vi "STD Cal Data_etc_old.vi"(8 "error in":errorcluster caption="에러 입력(에러 없음)", 9 "Data in":string[][](array[string]), 10 "문자열":string, 11 "Func_ext":string) -> (0 "error out":errorcluster caption="에러 출력", 1 "Data Out":string[][](array[string]), 3 "Func_ext Out":string, 4 "Data Out 2":string[](array[string]), 6 "Cal STD":string[][](array[string]))   [LabVIEW 2020]
uses:
  Support/Controls/Cmd_Var Data IO.ctl
  Support/Controls/Cmd_File path.ctl
  Support/Controls/Cmd_File Type.ctl
  Variables/Global_Cal STD.vi
  Variables/Global_Cal Info.vi
  Support/Public/Polymorph/Data Class_2D Str.vi
  Support/Public/Polymorph/Sort_2D Str.vi
  Support/Public/Polymorph/Array Dedup_2D Str.vi
  <vilib>/Utility/file.llb/Read Delimited Spreadsheet (string).vi
  Support/Public/Polymorph/Array Dedup_1D Str.vi
panel:
  out "Cal STD in":string[][](array[string])
  out "Condition Default":string[][](array[string])
  out "데이터오류?":bool
  out "생성오류?":bool
  out "Condition":string[][](array[string])
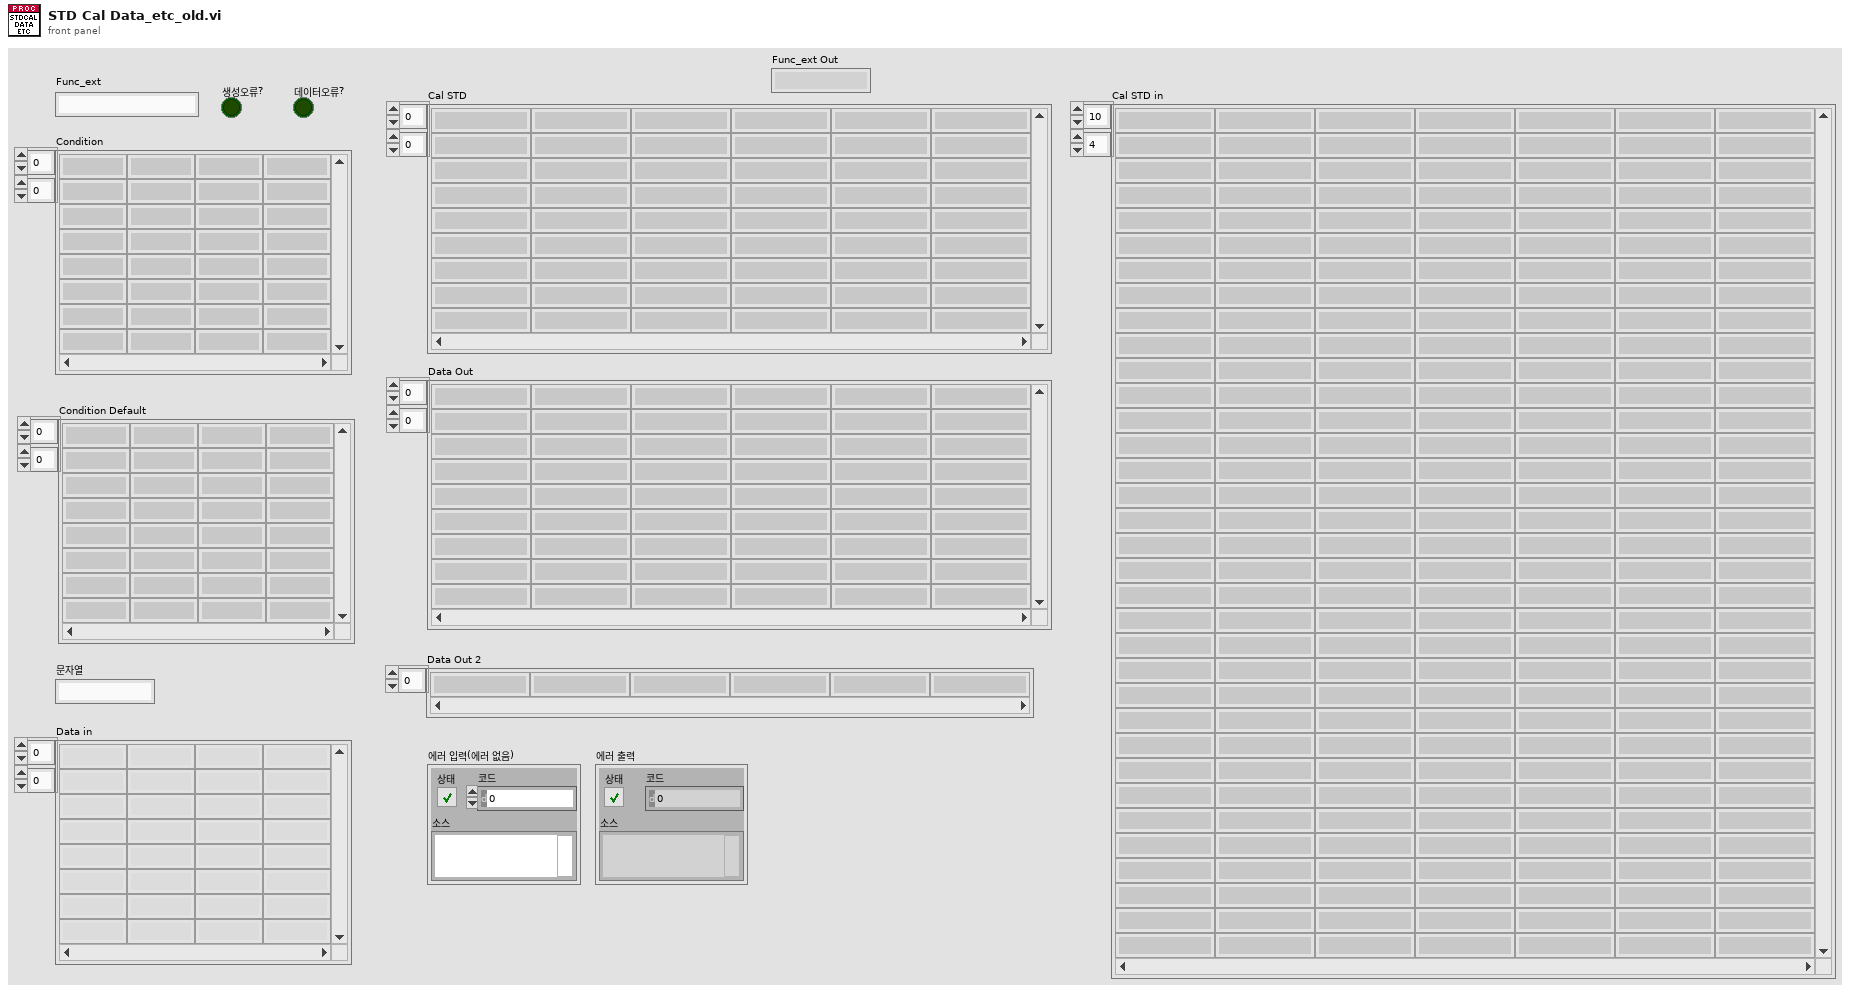
[diagram p1: front panel]
types:
  T1 = typedef "Cmd_Var Data IO.ctl" = enum16{"Condition", "Condition Default", "Condition_Temp", "Resolution", "Resolution Default", "Resolution Old", "Spec", "Spec Default", "Spec Old", "Spec Temp", "Result", "Result2", "Result3", "Result_Temp", "Result_ADJ", "Result_ADJ2", "STD1", "STD2", "STD3", "STD4", "STD5", "STD Temp", "CMC", "CMC Default"}
  T2 = cluster{"세부분류코드":string, "형식":string, "옵션":string, "측정기명":string, "EXCEL파일명":string, "TEMP":string}
  T3 = typedef "Cmd_File Type.ctl" = enum16{"엑셀", "엑셀(2003)", "텍스트", "설정", "2진", "VI", "CSV", "LOG", "폴더"}
  T4 = typedef "Cmd_File path.ctl" = enum16{"에러로그", "데이터파일경로", "성적서원본", "지난성적서", "Data Files", "경로생성", "Updater", "Template", "설정파일경로", "FTP Upload", "Update 경로", "어플리케이션"}
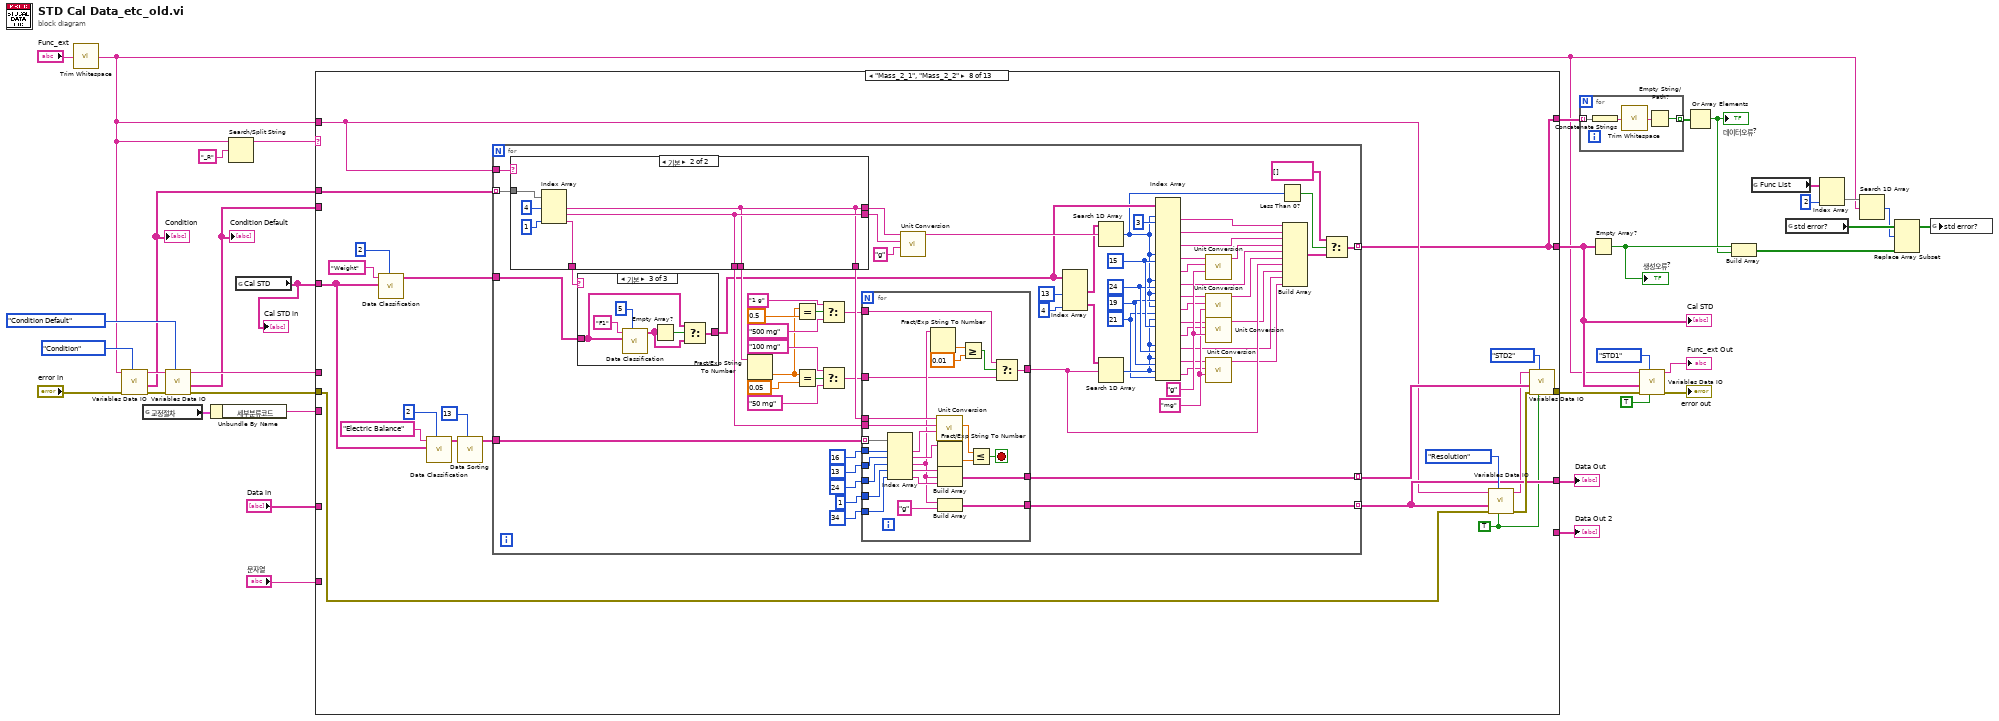
[diagram p0: block diagram]
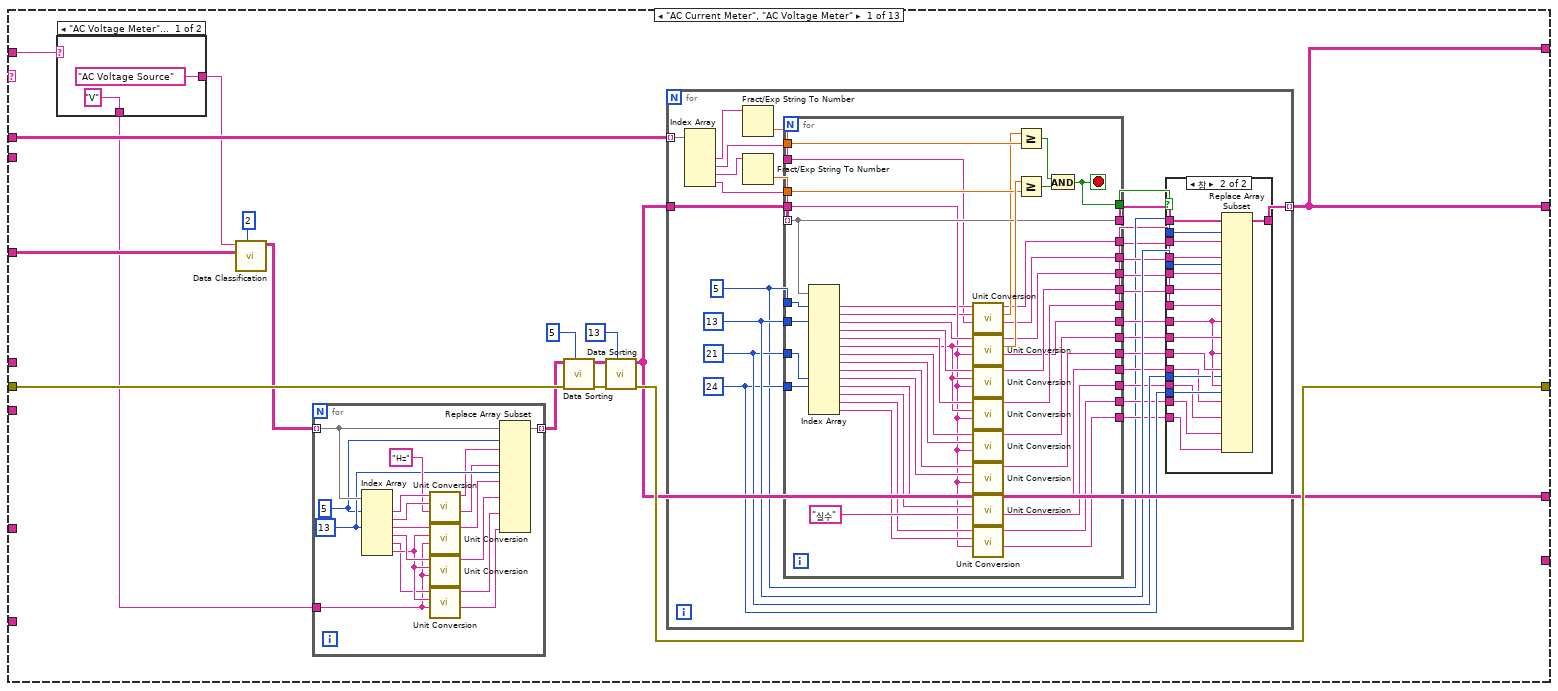
[diagram p2: hidden frame]
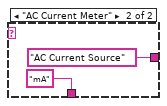
[diagram p3: hidden frame]
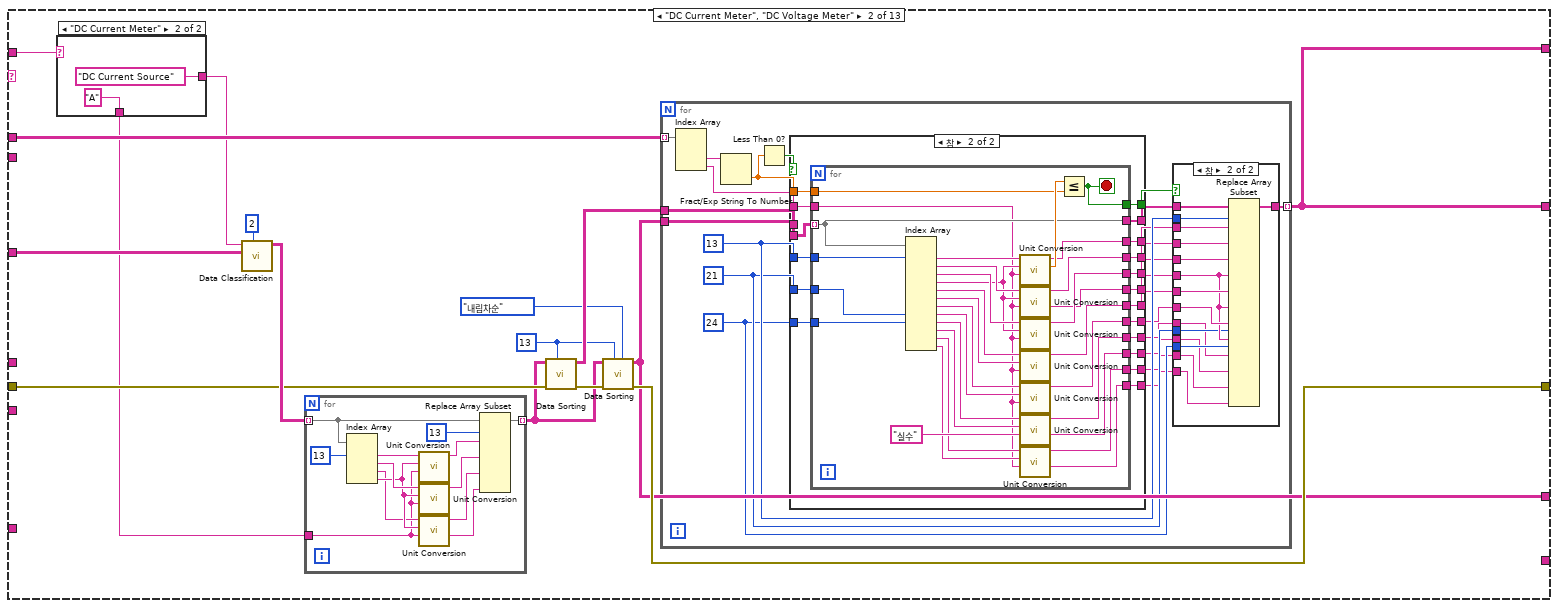
[diagram p5: hidden frame]
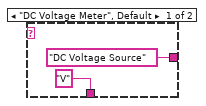
[diagram p6: hidden frame]
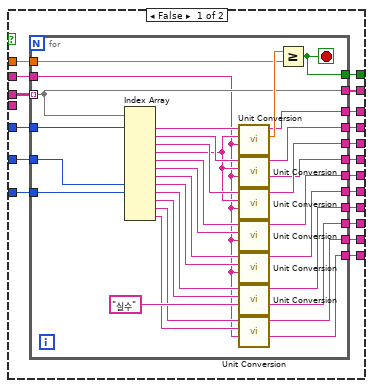
[diagram p8: hidden frame]
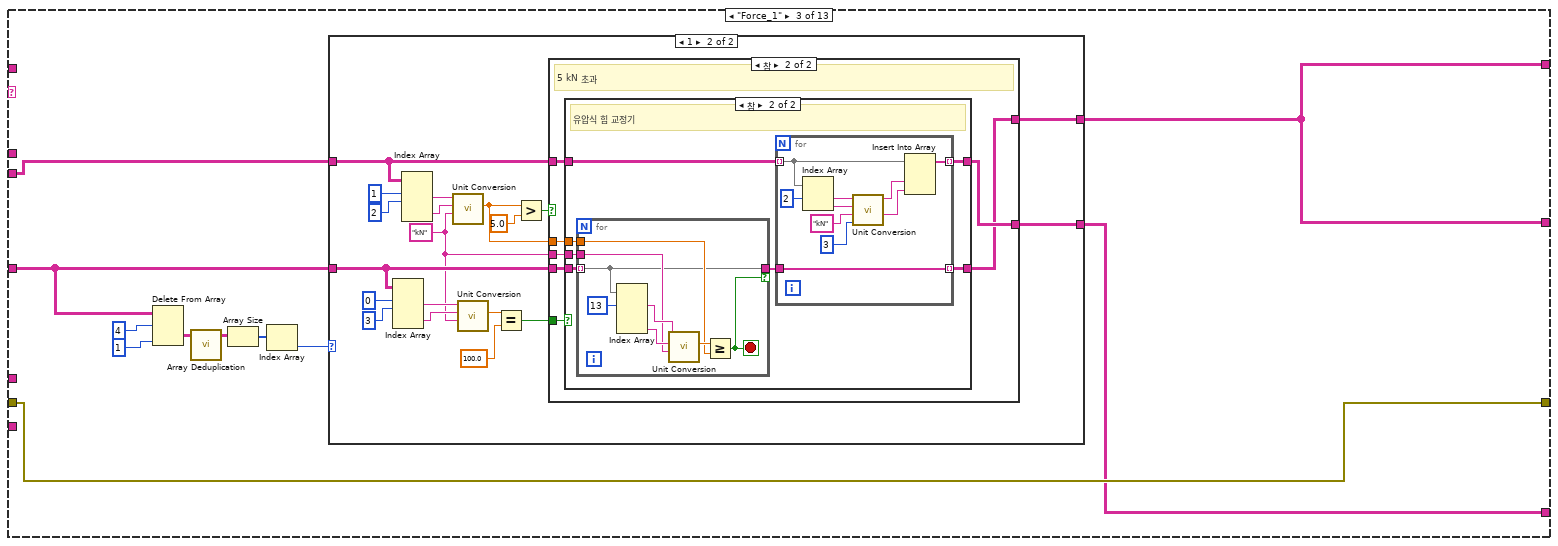
[diagram p9: hidden frame]
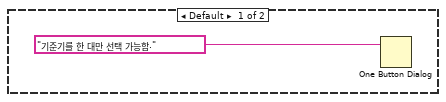
[diagram p10: hidden frame]
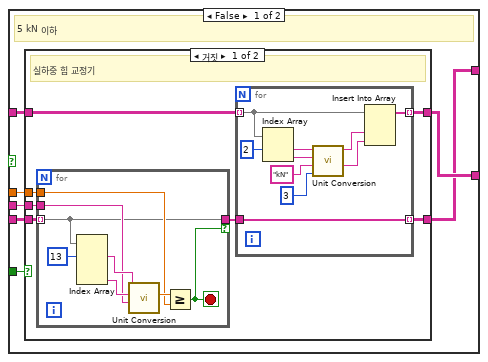
[diagram p11: hidden frame]
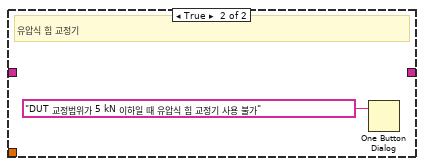
[diagram p12: hidden frame]
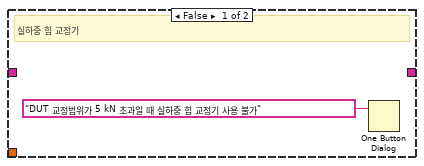
[diagram p13: hidden frame]
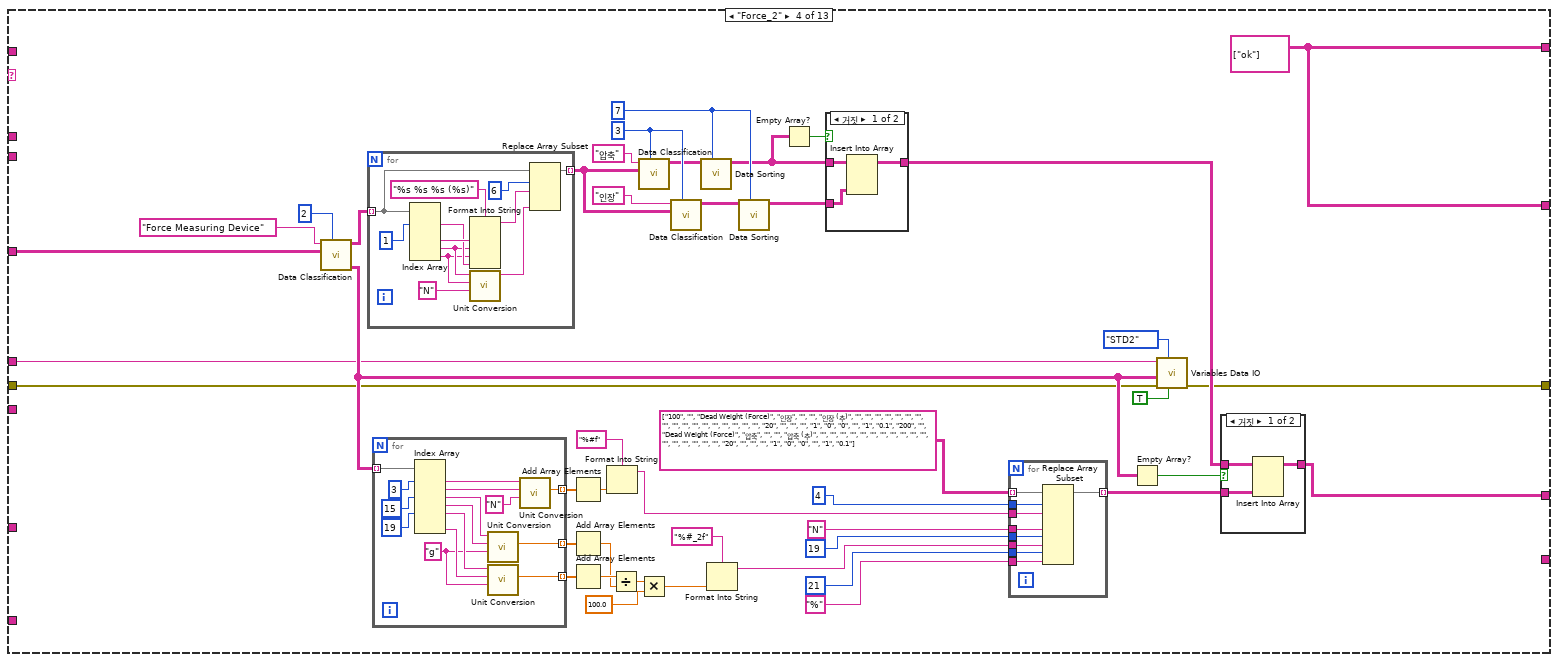
[diagram p14: hidden frame]
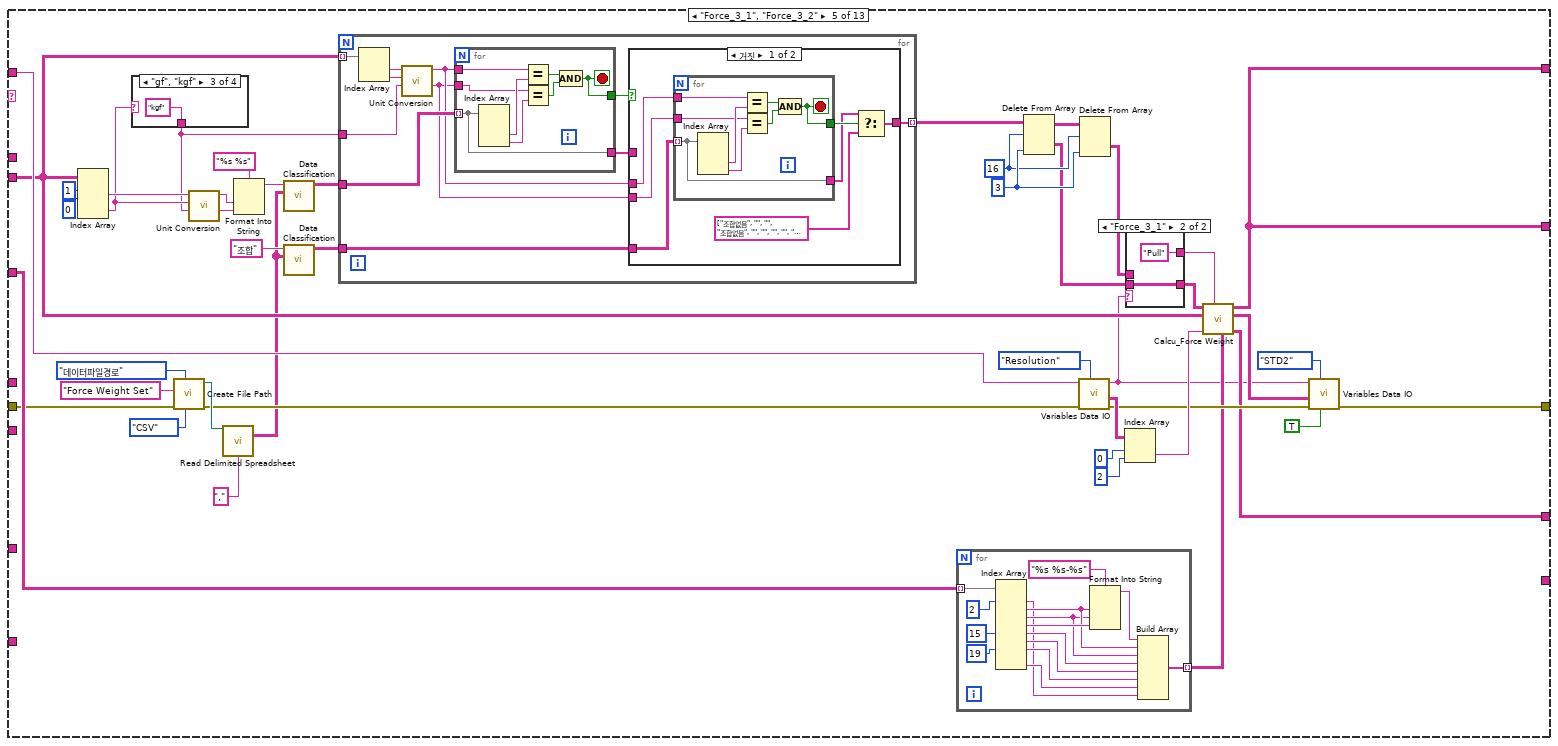
[diagram p17: hidden frame]
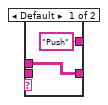
[diagram p18: hidden frame]
diagram:
  n1 = call <vilib>:"Trim Whitespace.vi"("string"="Func_ext") -> ("trimmed string"=w2:string)  [unwired: 1 in]
  n2 = call "Variables Data IO.vi"("Select"=Cmd_Var_Data_IO."Condition", "error in"="error in", "Func_ext"=w2) -> ("error out"=w24:errorcluster, "Data Out"=w9:string[][], "Func_ext Out"=w22:string)  [unwired: 6 in]
  "Condition" <- w9
  n3 = global read "Global_Cal Info.vi" "교정절차"() -> (w7:T2)
  n4 = call "Variables Data IO.vi"("Select"=Cmd_Var_Data_IO."Condition Default", "error in"=w24, "Func_ext"=w22) -> ("error out"=w23:errorcluster, "Data Out"=w8:string[][], "Func_ext Out"=w21:string)  [unwired: 6 in]
  "Condition Default" <- w8
  n5 = Unbundle By Name(w7) -> ("세부분류코드"=w6:string)
  n6 = Search/Split String(string=w2, search string/char (-)="_R" ("검색 문자열/문자 (-)")) -> (substring before match=w19:string)  [unwired: 1 in, 2 out]
  n7 = global read "Global_Cal STD.vi" "Cal STD"() -> (w37:string[][])
  "Cal STD in" <- w37
  n8 = case shown="\"Mass_2_1\", \"Mass_2_2\"" w19 {
    selector: w19 -> [_ _ _ _ _ _ _ _ w978 _ _ _ _]
    tunnel: w23 -> [w48 w174 w341 w442 w517 w628 w718 w852 w986 w1923 w2014 w2127 w2155]
    tunnel: [w50 w170 w341 w447 w533 w626 w738 w853 w984 w1921 w2039 w2126 w2155] -> w36
    tunnel: w37 -> [w52 w176 w334 w463 w551 w629 w754 w856 w983 w1924 w2052 w2128 _]
    tunnel: [w39 w163 w340 w449 w526 w619 w733 w836 w987 w1914 w2033 w2129 w2154] -> w27
    tunnel: [w40 w166 w338 w456 w527 w620 w723 w849 w980 w1915 w2029 w2128 _] -> w33
    tunnel: w9 -> [w51 w173 _ _ _ w627 w713 w847 _ w1922 _ _ _]
    tunnel: [w39 w163 w340 w449 w526 w619 w731 w836 w987 w1914 w2033 w2129 w2154] -> w26
    tunnel: w8 -> [_ _ w339 _ w542 _ _ _ w982 _ w2055 w2125 _]
    tunnel: w21 -> [_ _ _ w445 _ _ _ _ w985 _ w2028 w2124 _]
    tunnel: w2 -> [w38 w162 _ _ w547 w618 w722 w845 _ w1913 _ _ _]
    tunnel: w6 -> [_ _ _ _ _ _ _ _ w981 _ _ _ _]
    tunnel: [_ _ _ _ _ _ _ _ w979 _ _ _ string[] []] -> w5
    tunnel: "Data in" -> [_ _ _ _ _ _ _ _ w976 _ _ _ _]
    tunnel: "문자열" -> [_ _ _ _ _ _ _ _ w977 _ _ _ _]
    frame "AC Current Meter", "AC Voltage Meter" {
      n9 = case shown="\"AC Voltage Meter\", 기본" w38 {
        tunnel: ["AC Voltage Source" "AC Current Source"] -> w42
        tunnel: ["V" ("환산단위") "mA" ("환산단위")] -> w41
        frame "AC Voltage Meter", Default {
        }
        frame "AC Current Meter" {
        }
      }
      n10 = call-poly "Data Classification.vi"("인덱스"=2, "DATA 입력"=w52, "검색 문자열"=w42) -> ("DATA 출력"=w44:string[][])  [unwired: 4 in, 4 out]
      n11 = for {
        tunnel: w44 -> [w160] mode=indexing
        tunnel: [w156] -> w43 mode=indexing
        tunnel: w41 -> [w144]
        w147 = 5 ("인덱스")
        w148 = 13 ("인덱스")
        n12 = Index Array(array=w160, index #1=w147, index #3=w148) -> (element #1=w151:string, element #2=w150:string, element #3=w161:string, element #4=w159:string, element #5=w157:string, element #6=w158:string)  [unwired: 4 in]
        n13 = call "Unit Conversion.vi"("환산단위"="Hz", "입력단위"=w150, "입력값"=w151) -> ("환산단위"=w145:string, "환산값 (string)"=w146:string)  [unwired: 3 in, 4 out]
        n14 = call "Unit Conversion.vi"("환산단위"=w144, "입력단위"=w158, "입력값"=w161) -> ("환산값 (string)"=w155:string)  [unwired: 3 in, 5 out]
        n15 = call "Unit Conversion.vi"("환산단위"=w144, "입력단위"=w158, "입력값"=w159) -> ("환산값 (string)"=w154:string)  [unwired: 3 in, 5 out]
        n16 = call "Unit Conversion.vi"("환산단위"=w144, "입력단위"=w158, "입력값"=w157) -> ("환산단위"=w152:string, "환산값 (string)"=w153:string)  [unwired: 3 in, 4 out]
        n17 = Replace Array Subset(array=w160, new element #1=w146, index #1=w147, new element #2=w145, new element #3=w155, index #3=w148, new element #4=w154, new element #5=w153, new element #6=w152) -> (w156:string[])  [unwired: 4 in]
      }
      n18 = call-poly "Data Sorting.vi"("기준열"=u16 5, "error in (no error)"=w48, "Data in"=w43) -> ("error out"=w47:errorcluster, "Data out"=w46:string[][])  [unwired: 7 in]
      n19 = call-poly "Data Sorting.vi"("기준열"=u16 13, "error in (no error)"=w47, "Data in"=w46) -> ("error out"=w50:errorcluster, "Data out"=w40:string[][])  [unwired: 7 in]
      n20 = for {
        tunnel: w40 -> [w84]
        tunnel: w51 -> [w83] mode=indexing
        tunnel: [w77] -> w39 mode=indexing
        w60 = 5 ("인덱스")
        w74 = 24 ("인덱스")
        w75 = 21 ("인덱스")
        w76 = 13 ("인덱스")
        n21 = Index Array(array=w83) -> (element #2=w63:string, element #3=w61:string, element #4=w80:string, element #5=w82:string)  [unwired: 5 in, 1 out]
        n22 = Fract/Exp String To Number(string=w63) -> (number=w62:dbl)  [unwired: 3 in, 1 out]
        n23 = Fract/Exp String To Number(string=w80) -> (number=w81:dbl)  [unwired: 3 in, 1 out]
        n24 = for {
          tunnel: w84 -> [w108] mode=indexing
          tunnel: w82 -> [w96]
          tunnel: [w108] -> w78
          tunnel: w81 -> [w123]
          tunnel: w76 -> [w107]
          tunnel: w75 -> [w110]
          tunnel: w74 -> [w109]
          tunnel: [w85] -> w79
          tunnel: [w106] -> w73
          tunnel: [w105] -> w72
          tunnel: [w104] -> w71
          tunnel: [w103] -> w70
          tunnel: [w102] -> w69
          tunnel: [w101] -> w68
          tunnel: [w100] -> w67
          tunnel: [w99] -> w66
          tunnel: [w98] -> w65
          tunnel: [w97] -> w64
          tunnel: w62 -> [w92]
          tunnel: w60 -> [w95]
          tunnel: w61 -> [w90]
          tunnel: [w89] -> w59
          tunnel: [w88] -> w58
          stop <- w85 stop-if-true
          n25 = Index Array(array=w108, index #1=w95, index #3=w107, index #10=w110, index #11=w109) -> (element #1=w94:string, element #2=w93:string, element #3=w125:string, element #4=w122:string, element #5=w121:string, element #6=w120:string, element #7=w119:string, element #8=w118:string, element #9=w117:string, element #10=w116:string, element #11=w115:string, element #12=w114:string, element #13=w112:string, element #14=w111:string)  [unwired: 10 in]
          n26 = call "Unit Conversion.vi"("환산단위"=w90, "입력단위"=w93, "입력값"=w94) -> ("환산단위"=w88:string, "환산값 (DBL)"=w91:dbl, "환산값 (string)"=w89:string)  [unwired: 3 in, 3 out]
          n27 = call "Unit Conversion.vi"("환산단위"=w96, "입력단위"=w120, "입력값"=w125) -> ("환산단위"=w103:string, "환산값 (DBL)"=w124:dbl, "환산값 (string)"=w106:string)  [unwired: 3 in, 3 out]
          n28 = call "Unit Conversion.vi"("환산단위"=w96, "입력단위"=w120, "입력값"=w122) -> ("환산값 (string)"=w105:string)  [unwired: 3 in, 5 out]
          n29 = call "Unit Conversion.vi"("환산단위"=w96, "입력단위"=w120, "입력값"=w121) -> ("환산값 (string)"=w104:string)  [unwired: 3 in, 5 out]
          n30 = call "Unit Conversion.vi"("환산단위"=w96, "입력단위"=w118, "입력값"=w119) -> ("환산값 (string)"=w102:string)  [unwired: 3 in, 5 out]
          n31 = call "Unit Conversion.vi"("환산단위"=w96, "입력단위"=w116, "입력값"=w117) -> ("환산값 (string)"=w101:string)  [unwired: 3 in, 5 out]
          n32 = call "Unit Conversion.vi"("환산단위"="실수", "입력단위"=w114, "입력값"=w115) -> ("환산단위"=w99:string, "환산값 (string)"=w100:string)  [unwired: 3 in, 4 out]
          n33 = call "Unit Conversion.vi"("환산단위"=w96, "입력단위"=w111, "입력값"=w112) -> ("환산단위"=w97:string, "환산값 (string)"=w98:string)  [unwired: 3 in, 4 out]
          n34 = Greater Or Equal?(x=w91, y=w92) -> (x >= y?=w87:bool)
          n35 = Greater Or Equal?(x=w124, y=w123) -> (x >= y?=w86:bool)
          n36 = And(x=w87, y=w86) -> (x .and. y?=w85:bool)
        }
        n37 = case shown="참" w79 {
          tunnel: w78 -> [_ w143]
          tunnel: [_ w142] -> w77
          tunnel: w76 -> [_ w141]
          tunnel: w73 -> [_ w140]
          tunnel: w72 -> [_ w139]
          tunnel: w71 -> [_ w138]
          tunnel: w70 -> [_ w135]
          tunnel: w69 -> [_ w137]
          tunnel: w68 -> [_ w136]
          tunnel: w67 -> [_ w132]
          tunnel: w75 -> [_ w134]
          tunnel: w66 -> [_ w131]
          tunnel: w74 -> [_ w133]
          tunnel: w65 -> [_ w130]
          tunnel: w64 -> [_ w129]
          tunnel: w60 -> [_ w128]
          tunnel: w59 -> [_ w127]
          tunnel: w58 -> [_ w126]
          frame False {
          }
          frame True {
            n38 = Replace Array Subset(array=w143, new element #1=w127, index #1=w128, new element #2=w126, new element #3=w140, index #3=w141, new element #4=w139, new element #5=w138, new element #6=w135, new element #7=w137, new element #8=w135, new element #9=w136, new element #10=w135, index #10=w134, new element #11=w132, index #11=w133, new element #12=w131, new element #13=w130, new element #14=w129) -> (w142:string[])  [unwired: 10 in]
          }
        }
      }
    }
    frame "DC Current Meter", "DC Voltage Meter" {
      w168 = u16 13 ("기준열")
      n39 = case shown="\"DC Current Meter\"" w162 {
        tunnel: ["DC Voltage Source" "DC Current Source"] -> w165
        tunnel: ["V" ("환산단위") "A" ("환산단위")] -> w164
        frame "DC Voltage Meter", Default {
        }
        frame "DC Current Meter" {
        }
      }
      n40 = call-poly "Data Classification.vi"("인덱스"=2, "DATA 입력"=w176, "검색 문자열"=w165) -> ("DATA 출력"=w175:string[][])  [unwired: 4 in, 4 out]
      n41 = for {
        tunnel: w175 -> [w328] mode=indexing
        tunnel: [w323] -> w169 mode=indexing
        tunnel: w164 -> [w318]
        n42 = Index Array(array=w328, index #1=13 ("인덱스")) -> (element #1=w329:string, element #2=w327:string, element #3=w325:string, element #4=w326:string)  [unwired: 3 in]
        n43 = call "Unit Conversion.vi"("환산단위"=w318, "입력단위"=w326, "입력값"=w329) -> ("환산값 (string)"=w322:string)  [unwired: 3 in, 5 out]
        n44 = call "Unit Conversion.vi"("환산단위"=w318, "입력단위"=w326, "입력값"=w327) -> ("환산값 (string)"=w321:string)  [unwired: 3 in, 5 out]
        n45 = call "Unit Conversion.vi"("환산단위"=w318, "입력단위"=w326, "입력값"=w325) -> ("환산단위"=w319:string, "환산값 (string)"=w320:string)  [unwired: 3 in, 4 out]
        n46 = Replace Array Subset(array=w328, new element #1=w322, index #1=13 ("인덱스"), new element #2=w321, new element #3=w320, new element #4=w319) -> (w323:string[])  [unwired: 3 in]
      }
      n47 = call-poly "Data Sorting.vi"("기준열"=w168, "error in (no error)"=w174, "Data in"=w169) -> ("error out"=w171:errorcluster, "Data out"=w172:string[][])  [unwired: 7 in]
      n48 = call-poly "Data Sorting.vi"("정렬"=enum16{"오름차순", "내림차순"}."내림차순", "기준열"=w168, "error in (no error)"=w171, "Data in"=w169) -> ("error out"=w170:errorcluster, "Data out"=w166:string[][])  [unwired: 6 in]
      n49 = for {
        tunnel: w172 -> [w204]
        tunnel: w173 -> [w203] mode=indexing
        tunnel: [w195] -> w163 mode=indexing
        tunnel: w166 -> [w199]
        w192 = 24 ("인덱스")
        w193 = 21 ("인덱스")
        w194 = 13 ("인덱스")
        n50 = Index Array(array=w203) -> (element #2=w198:string, element #3=w202:string)  [unwired: 3 in, 1 out]
        n51 = Fract/Exp String To Number(string=w198) -> (number=w201:dbl)  [unwired: 3 in, 1 out]
        n52 = Less Than 0?(x=w201) -> (x < 0?=w200:bool)
        n53 = case shown="참" w200 {
          tunnel: w204 -> [w237 _]
          tunnel: w202 -> [w236 w286]
          tunnel: [w235 w285] -> w196
          tunnel: w201 -> [w234 w284]
          tunnel: w199 -> [_ w269]
          tunnel: w194 -> [w233 w283]
          tunnel: w193 -> [w232 w282]
          tunnel: w192 -> [w231 w281]
          tunnel: [w230 w280] -> w197
          tunnel: [w229 w279] -> w191
          tunnel: [w228 w278] -> w190
          tunnel: [w227 w277] -> w189
          tunnel: [w226 w276] -> w188
          tunnel: [w225 w275] -> w187
          tunnel: [w224 w274] -> w186
          tunnel: [w223 w273] -> w185
          tunnel: [w222 w272] -> w184
          tunnel: [w221 w271] -> w183
          tunnel: [w220 w270] -> w182
          frame False {
            n54 = for {
              tunnel: w237 -> [w250] mode=indexing
              tunnel: w236 -> [w239]
              tunnel: [w250] -> w235
              tunnel: w234 -> [w266]
              tunnel: w233 -> [w249]
              tunnel: w232 -> [w253]
              tunnel: w231 -> [w252]
              tunnel: [w251] -> w230
              tunnel: [w248] -> w229
              tunnel: [w247] -> w228
              tunnel: [w246] -> w227
              tunnel: [w238] -> w226
              tunnel: [w245] -> w225
              tunnel: [w244] -> w224
              tunnel: [w243] -> w223
              tunnel: [w242] -> w222
              tunnel: [w241] -> w221
              tunnel: [w240] -> w220
              stop <- w251 stop-if-true
              n55 = Index Array(array=w250, index #1=w249, index #8=w253, index #9=w252) -> (element #1=w268:string, element #2=w265:string, element #3=w264:string, element #4=w263:string, element #5=w262:string, element #6=w261:string, element #7=w260:string, element #8=w259:string, element #9=w258:string, element #10=w257:string, element #11=w255:string, element #12=w254:string)  [unwired: 9 in]
              n56 = call "Unit Conversion.vi"("환산단위"=w239, "입력단위"=w263, "입력값"=w268) -> ("환산값 (DBL)"=w267:dbl, "환산값 (string)"=w248:string)  [unwired: 3 in, 4 out]
              n57 = call "Unit Conversion.vi"("환산단위"=w239, "입력단위"=w263, "입력값"=w265) -> ("환산단위"=w238:string, "환산값 (string)"=w247:string)  [unwired: 3 in, 4 out]
              n58 = call "Unit Conversion.vi"("환산단위"=w239, "입력단위"=w263, "입력값"=w264) -> ("환산값 (string)"=w246:string)  [unwired: 3 in, 5 out]
              n59 = call "Unit Conversion.vi"("환산단위"=w239, "입력단위"=w261, "입력값"=w262) -> ("환산값 (string)"=w245:string)  [unwired: 3 in, 5 out]
              n60 = call "Unit Conversion.vi"("환산단위"=w239, "입력단위"=w259, "입력값"=w260) -> ("환산값 (string)"=w244:string)  [unwired: 3 in, 5 out]
              n61 = call "Unit Conversion.vi"("환산단위"="실수", "입력단위"=w257, "입력값"=w258) -> ("환산단위"=w242:string, "환산값 (string)"=w243:string)  [unwired: 3 in, 4 out]
              n62 = call "Unit Conversion.vi"("환산단위"=w239, "입력단위"=w254, "입력값"=w255) -> ("환산단위"=w240:string, "환산값 (string)"=w241:string)  [unwired: 3 in, 4 out]
              n63 = Greater Or Equal?(x=w267, y=w266) -> (x >= y?=w251:bool)
            }
          }
          frame True {
            n64 = for {
              tunnel: w269 -> [w299] mode=indexing
              tunnel: w286 -> [w288]
              tunnel: [w299] -> w285
              tunnel: w284 -> [w315]
              tunnel: w283 -> [w298]
              tunnel: w282 -> [w302]
              tunnel: w281 -> [w301]
              tunnel: [w300] -> w280
              tunnel: [w297] -> w279
              tunnel: [w296] -> w278
              tunnel: [w295] -> w277
              tunnel: [w287] -> w276
              tunnel: [w294] -> w275
              tunnel: [w293] -> w274
              tunnel: [w292] -> w273
              tunnel: [w291] -> w272
              tunnel: [w290] -> w271
              tunnel: [w289] -> w270
              stop <- w300 stop-if-true
              n65 = Index Array(array=w299, index #1=w298, index #8=w302, index #9=w301) -> (element #1=w317:string, element #2=w314:string, element #3=w313:string, element #4=w312:string, element #5=w311:string, element #6=w310:string, element #7=w309:string, element #8=w308:string, element #9=w307:string, element #10=w306:string, element #11=w304:string, element #12=w303:string)  [unwired: 9 in]
              n66 = call "Unit Conversion.vi"("환산단위"=w288, "입력단위"=w312, "입력값"=w317) -> ("환산값 (DBL)"=w316:dbl, "환산값 (string)"=w297:string)  [unwired: 3 in, 4 out]
              n67 = call "Unit Conversion.vi"("환산단위"=w288, "입력단위"=w312, "입력값"=w314) -> ("환산단위"=w287:string, "환산값 (string)"=w296:string)  [unwired: 3 in, 4 out]
              n68 = call "Unit Conversion.vi"("환산단위"=w288, "입력단위"=w312, "입력값"=w313) -> ("환산값 (string)"=w295:string)  [unwired: 3 in, 5 out]
              n69 = call "Unit Conversion.vi"("환산단위"=w288, "입력단위"=w310, "입력값"=w311) -> ("환산값 (string)"=w294:string)  [unwired: 3 in, 5 out]
              n70 = call "Unit Conversion.vi"("환산단위"=w288, "입력단위"=w308, "입력값"=w309) -> ("환산값 (string)"=w293:string)  [unwired: 3 in, 5 out]
              n71 = call "Unit Conversion.vi"("환산단위"="실수", "입력단위"=w306, "입력값"=w307) -> ("환산단위"=w291:string, "환산값 (string)"=w292:string)  [unwired: 3 in, 4 out]
              n72 = call "Unit Conversion.vi"("환산단위"=w288, "입력단위"=w303, "입력값"=w304) -> ("환산단위"=w289:string, "환산값 (string)"=w290:string)  [unwired: 3 in, 4 out]
              n73 = Less Or Equal?(x=w316, y=w315) -> (x <= y?=w300:bool)
            }
          }
        }
        n74 = case shown="참" w197 {
          tunnel: w196 -> [_ w219]
          tunnel: [_ w218] -> w195
          tunnel: w194 -> [_ w217]
          tunnel: w191 -> [_ w216]
          tunnel: w190 -> [_ w215]
          tunnel: w189 -> [_ w214]
          tunnel: w188 -> [_ w211]
          tunnel: w187 -> [_ w213]
          tunnel: w186 -> [_ w212]
          tunnel: w185 -> [_ w208]
          tunnel: w193 -> [_ w210]
          tunnel: w184 -> [_ w207]
          tunnel: w192 -> [_ w209]
          tunnel: w183 -> [_ w206]
          tunnel: w182 -> [_ w205]
          frame False {
          }
          frame True {
            n75 = Replace Array Subset(array=w219, new element #1=w216, index #1=w217, new element #2=w215, new element #3=w214, new element #4=w211, new element #5=w213, new element #6=w211, new element #7=w212, new element #8=w211, index #8=w210, new element #9=w208, index #9=w209, new element #10=w207, new element #11=w206, new element #12=w205) -> (w218:string[])  [unwired: 9 in]
          }
        }
      }
    }
    frame "Force_1" {
      n76 = Delete From Array(array=w334, length=4 ("길이"), index (col)=1 ("비활성화된 인덱스 (열)")) -> (deleted portion=w333:string[][])  [unwired: 1 in, 1 out]
      n77 = call-poly "Array Deduplication.vi"("배열 in"=w333) -> ("배열 out"=w335:string[][])  [unwired: 9 in, 1 out]
      n78 = Array Size(array=w335) -> (size(s)=w337:i32[])
      n79 = Index Array(array=w337) -> (element=w336:i32)  [unwired: 1 in]
      n80 = case shown="1" w336 {
        tunnel: [_ w361] -> w340
        tunnel: w339 -> [_ w360]
        tunnel: w334 -> [_ w351]
        tunnel: [_ w346] -> w338
        frame Default {
          n81 = One Button Dialog(message="기준기를 한 대만 선택 가능함.") -> ()  [unwired: 1 in, 1 out]
        }
        frame 1 {
          w347 = "kN" ("환산단위")
          n82 = Index Array(array=w351, index (row) #1=0 ("비활성화된 인덱스 (행)"), index (col) #1=3 ("비활성화된 인덱스 (열)")) -> (element #1=w349:string, element #2=w350:string)  [unwired: 2 in]
          n83 = Index Array(array=w360, index (row) #1=1 ("인덱스 (행)"), index (col) #1=2 ("비활성화된 인덱스 (열)")) -> (element #1=w357:string, element #2=w356:string)  [unwired: 2 in]
          n84 = call "Unit Conversion.vi"("환산단위"=w347, "입력단위"=w356, "입력값"=w357) -> ("환산값 (DBL)"=w348:dbl)  [unwired: 3 in, 5 out]
          n85 = call "Unit Conversion.vi"("환산단위"=w347, "입력단위"=w350, "입력값"=w349) -> ("환산값 (DBL)"=w345:dbl)  [unwired: 3 in, 5 out]
          n86 = Equal?(x=w345, y=100.0) -> (x = y?=w343:bool)
          n87 = Greater?(x=w348, y=5.0) -> (0:w354:bool)
          n88 = case shown="참" w354 {
            tunnel: [w363 w396] -> w361
            tunnel: w360 -> [w368 w401]
            tunnel: w351 -> [w367 w400]
            tunnel: w348 -> [w366 w399]
            tunnel: w347 -> [w365 w398]
            tunnel: [w364 w397] -> w346
            tunnel: w343 -> [w362 w395]
            frame False {
              # "5 kN 이하"
              n89 = case shown="거짓" w362 {
                tunnel: [w375 _] -> w364
                tunnel: w368 -> [w374 _]
                tunnel: w367 -> [w373 _]
                tunnel: w366 -> [w372 _]
                tunnel: w365 -> [w371 _]
                tunnel: [w369 _] -> w363
                frame False {
                  # "실하중 힘 교정기"
                  n90 = for {
                    tunnel: w373 -> [w377] mode=indexing
                    tunnel: w372 -> [w378]
                    tunnel: w371 -> [w380]
                    tunnel: [w377] -> w370 if=w376
                    stop <- w376 stop-if-true
                    n91 = Index Array(array=w377, index #1=13 ("인덱스")) -> (element #1=w382:string, element #4=w381:string)  [unwired: 3 in, 2 out]
                    n92 = call "Unit Conversion.vi"("환산단위"=w380, "입력단위"=w381, "입력값"=w382) -> ("환산값 (DBL)"=w379:dbl)  [unwired: 3 in, 5 out]
                    n93 = Greater Or Equal?(x=w379, y=w378) -> (x >= y?=w376:bool)
                  }
                  n94 = for {
                    tunnel: w374 -> [w393] mode=indexing
                    tunnel: [w390] -> w375 mode=indexing
                    tunnel: w370 -> [w388]
                    tunnel: [w388] -> w369 mode=indexing
                    n95 = Index Array(array=w393, index #1=2 ("인덱스")) -> (element #1=w389:string, element #2=w386:string)  [unwired: 1 in]
                    n96 = call "Unit Conversion.vi"("소수점 자리수"=3, "환산단위"="kN", "입력단위"=w386, "입력값"=w389) -> ("환산단위"=w391:string, "환산값 (string)"=w392:string)  [unwired: 2 in, 4 out]
                    n97 = Insert Into Array(array=w393, new element #1=w392, new element #2=w391) -> (w390:string[])  [unwired: 1 in]
                  }
                }
                frame True {
                  # "유압식 힘 교정기"
                  n98 = One Button Dialog(message="DUT 교정범위가 5 kN 이하일 때 유압식 힘 교정기 사용 불가") -> ()  [unwired: 1 in, 1 out]
                }
              }
            }
            frame True {
              # "5 kN 초과"
              n99 = case shown="참" w395 {
                tunnel: [_ w409] -> w397
                tunnel: w401 -> [_ w408]
                tunnel: w400 -> [_ w407]
                tunnel: w399 -> [_ w406]
                tunnel: w398 -> [_ w405]
                tunnel: [_ w403] -> w396
                frame False {
                  # "실하중 힘 교정기"
                  n100 = One Button Dialog(message="DUT 교정범위가 5 kN 초과일 때 실하중 힘 교정기 사용 불가") -> ()  [unwired: 1 in, 1 out]
                }
                frame True {
                  # "유압식 힘 교정기"
                  n101 = for {
                    tunnel: w407 -> [w411] mode=indexing
                    tunnel: w406 -> [w412]
                    tunnel: w405 -> [w414]
                    tunnel: [w411] -> w404 if=w410
                    stop <- w410 stop-if-true
                    n102 = Index Array(array=w411, index #1=13 ("인덱스")) -> (element #1=w416:string, element #4=w415:string)  [unwired: 3 in, 2 out]
                    n103 = call "Unit Conversion.vi"("환산단위"=w414, "입력단위"=w415, "입력값"=w416) -> ("환산값 (DBL)"=w413:dbl)  [unwired: 3 in, 5 out]
                    n104 = Greater Or Equal?(x=w413, y=w412) -> (x >= y?=w410:bool)
                  }
                  n105 = for {
                    tunnel: w408 -> [w427] mode=indexing
                    tunnel: [w424] -> w409 mode=indexing
                    tunnel: w404 -> [w422]
                    tunnel: [w422] -> w403 mode=indexing
                    n106 = Index Array(array=w427, index #1=2 ("인덱스")) -> (element #1=w423:string, element #2=w420:string)  [unwired: 1 in]
                    n107 = call "Unit Conversion.vi"("소수점 자리수"=3, "환산단위"="kN", "입력단위"=w420, "입력값"=w423) -> ("환산단위"=w425:string, "환산값 (string)"=w426:string)  [unwired: 2 in, 4 out]
                    n108 = Insert Into Array(array=w427, new element #1=w426, new element #2=w425) -> (w424:string[])  [unwired: 1 in]
                  }
                }
              }
            }
          }
        }
      }
    }
    frame "Force_2" {
      w470 = 3 ("인덱스")
      w471 = u16 7 ("기준열")
      w449 = string[][] [["ok"]] ("Data out")
      n109 = call-poly "Data Classification.vi"("인덱스"=2, "DATA 입력"=w463, "검색 문자열"="Force Measuring Device") -> ("제외 DATA 출력"=w446:string[][], "DATA 출력"=w462:string[][])  [unwired: 4 in, 3 out]
      n110 = for {
        tunnel: w462 -> [w513] mode=indexing
        tunnel: [w510] -> w464 mode=indexing
        n111 = Index Array(array=w513, index #1=1 ("인덱스")) -> (element #1=w508:string, element #3=w515:string, element #4=w507:string, element #5=w506:string)  [unwired: 4 in, 1 out]
        n112 = Format Into String(format string="%s %s %s (%s)" ("포맷 문자열"), w515, w507, w506, w508) -> (resulting string=w511:string)  [unwired: 2 in, 1 out]
        n113 = call "Unit Conversion.vi"("환산단위"="N", "입력단위"=w506, "입력값"=w507) -> ("환산값 (string)"=w504:string)  [unwired: 3 in, 5 out]
        n114 = Replace Array Subset(array=w513, new element #1=w511, index #1=6 ("인덱스"), new element #2=w504) -> (w510:string[])  [unwired: 1 in]
      }
      n115 = for {
        tunnel: w446 -> [w494] mode=indexing
        tunnel: [w490] -> w455 mode=indexing
        tunnel: [w482] -> w441 mode=indexing
        tunnel: [w481] -> w440 mode=indexing
        w483 = "g" ("환산단위")
        n116 = Index Array(array=w494, index #1=3 ("인덱스"), index #3=15 ("인덱스"), index #5=19 ("인덱스")) -> (element #1=w492:string, element #2=w491:string, element #3=w488:string, element #4=w487:string, element #5=w485:string, element #7=w484:string)  [unwired: 4 in, 1 out]
        n117 = call "Unit Conversion.vi"("환산단위"=w483, "입력단위"=w487, "입력값"=w488) -> ("환산값 (DBL)"=w482:dbl)  [unwired: 3 in, 5 out]
        n118 = call "Unit Conversion.vi"("환산단위"=w483, "입력단위"=w484, "입력값"=w485) -> ("환산값 (DBL)"=w481:dbl)  [unwired: 3 in, 5 out]
        n119 = call "Unit Conversion.vi"("환산단위"="N", "입력단위"=w491, "입력값"=w492) -> ("환산값 (DBL)"=w490:dbl)  [unwired: 3 in, 5 out]
      }
      n120 = Add Array Elements(numeric array=w455) -> (sum=w454:dbl)
      n121 = Add Array Elements(numeric array=w441) -> (sum=w438:dbl)
      n122 = Add Array Elements(numeric array=w440) -> (sum=w439:dbl)
      n123 = Format Into String(format string="%#f" ("포맷 문자열"), w454) -> (resulting string=w452:string)  [unwired: 2 in, 1 out]
      n124 = Divide(x=w439, y=w438) -> (x/y=w437:dbl)
      n125 = call-poly "Data Classification.vi"("인덱스"=w470, "DATA 입력"=w464, "검색 문자열"="압축") -> ("DATA 출력"=w465:string[][])  [unwired: 4 in, 4 out]
      n126 = Multiply(x=w437, y=100.0) -> (x*y=w434:dbl)
      n127 = call-poly "Data Classification.vi"("인덱스"=w470, "DATA 입력"=w464, "검색 문자열"="인장") -> ("DATA 출력"=w468:string[][])  [unwired: 4 in, 4 out]
      n128 = call-poly "Data Sorting.vi"("기준열"=w471, "Data in"=w465) -> ("Data out"=w459:string[][])  [unwired: 8 in, 1 out]
      n129 = Format Into String(format string="%#_2f" ("포맷 문자열"), w434) -> (resulting string=w433:string)  [unwired: 2 in, 1 out]
      n130 = call-poly "Data Sorting.vi"("기준열"=w471, "Data in"=w468) -> ("Data out"=w469:string[][])  [unwired: 8 in, 1 out]
      n131 = Empty Array?(array=w459) -> (empty?=w458:bool)
      n132 = case shown="거짓" w458 {
        tunnel: w469 -> [w502 w503]
        tunnel: [w501 w503] -> w457
        tunnel: w459 -> [w500 _]
        frame False {
          n133 = Insert Into Array(array=w500, new element=w502) -> (w501:string[][])  [unwired: 2 in]
        }
        frame True {
        }
      }
      n134 = for {
        tunnel: string[][] [["100", "", "Dead Weight (Force)", "인장", "", "", "인장 (추)", "", "", "", "", "", "", "", "", "", "", "", "", "", "", "", "", "", "20", "", "", "", "1", "0", "0", "", "1", "0.1"], ["200", "", "Dead Weight (Force)", "압축", "", "", "압축 (추)", "", "", "", "", "", "", "", "", "", "", "", "", "", "", "", "", "", "20", "", "", "", "1", "0", "0", "", "1", "0.1"]] -> [w480] mode=indexing
        tunnel: w452 -> [w479]
        tunnel: [w478] -> w451 mode=indexing
        tunnel: "N" ("새 원소/부분배열") -> [w477]
        tunnel: 19 ("인덱스") -> [w476]
        tunnel: w433 -> [w475]
        tunnel: 21 ("인덱스") -> [w474]
        tunnel: "%" ("새 원소/부분배열") -> [w473]
        tunnel: 4 ("인덱스") -> [w472]
        n135 = Replace Array Subset(array=w480, new element #1=w479, index #1=w472, new element #2=w477, new element #3=w475, index #3=w476, new element #4=w473, index #4=w474) -> (w478:string[])  [unwired: 1 in]
      }
      n136 = Empty Array?(array=w446) -> (empty?=w444:bool)
      n137 = call "Variables Data IO.vi"("Write blank data ?(F)"=TRUE ("Write blank data ?(T)"), "Select"=Cmd_Var_Data_IO."STD2", "error in"=w442, "Data In"=w446, "Func_ext"=w445) -> ("error out"=w447:errorcluster)  [unwired: 4 in, 2 out]
      n138 = case shown="거짓" w444 {
        tunnel: [w498 w499] -> w456
        tunnel: w457 -> [w497 w499]
        tunnel: w451 -> [w496 _]
        frame False {
          n139 = Insert Into Array(array=w497, new element=w496) -> (w498:string[][])  [unwired: 2 in]
        }
        frame True {
        }
      }
    }
    frame "Force_3_1", "Force_3_2" {
      w538 = 16 ("길이")
      w539 = 3 ("비활성화된 인덱스 (열)")
      n140 = Index Array(array=w542, index (row) #1=1 ("인덱스 (행)"), index (col) #1=0 ("비활성화된 인덱스 (열)")) -> (element #1=w558:string, element #2=w557:string)  [unwired: 2 in]
      n141 = case shown="\"gf\", \"kgf\"" w557 {
        tunnel: [_ "N" "kgf" "lbf"] -> w550
        frame Default {
        }
        frame "N", "cN", "kN" {
        }
        frame "gf", "kgf" {
        }
        frame "lbf", "ozf" {
        }
      }
      n142 = call "Create File Path.vi"("파일타입"=Cmd_File_Type."CSV", "항목"=Cmd_File_path."데이터파일경로", "에러 입력"=w517, "문자열 in"="Force Weight Set" ("delimiter (\\t)")) -> ("error out"=w518:errorcluster, "파일경로"=w519:path)  [unwired: 4 in, 2 out]
      n143 = call "Unit Conversion.vi"("환산단위"=w550, "입력단위"=w557, "입력값"=w558) -> ("환산단위"=w555:string, "환산값 (string)"=w556:string)  [unwired: 3 in, 4 out]
      n144 = call-poly <vilib>:"Read Delimited Spreadsheet.vi"("file path (dialog if empty)"=w519, "delimiter (\\t)"="," ("delimiter (\\t)")) -> ("all rows"=w516:string[][])  [unwired: 8 in, 5 out]
      n145 = Format Into String(format string="%s %s" ("포맷 문자열"), w556, w555) -> (resulting string=w553:string)  [unwired: 2 in, 1 out]
      n146 = call-poly "Data Classification.vi"("DATA 입력"=w516, "검색 문자열"=w553) -> ("DATA 출력"=w523:string[][])  [unwired: 5 in, 4 out]
      n147 = call-poly "Data Classification.vi"("DATA 입력"=w516, "검색 문자열"="조합") -> ("DATA 출력"=w524:string[][])  [unwired: 5 in, 4 out]
      n148 = for {
        tunnel: w542 -> [w575] mode=indexing
        tunnel: w550 -> [w571]
        tunnel: w523 -> [w574]
        tunnel: w524 -> [w567]
        tunnel: [w568] -> w548 mode=indexing
        n149 = Index Array(array=w575) -> (element #1=w573:string, element #2=w572:string)  [unwired: 2 in]
        n150 = call "Unit Conversion.vi"("환산단위"=w571, "입력단위"=w572, "입력값"=w573) -> ("환산단위"=w565:string, "환산값 (string)"=w566:string)  [unwired: 3 in, 4 out]
        n151 = for {
          tunnel: w574 -> [w593] mode=indexing
          tunnel: w566 -> [w599]
          tunnel: w565 -> [w597]
          tunnel: [w593] -> w569
          tunnel: [w592] -> w570
          stop <- w592 stop-if-true
          n152 = Index Array(array=w593) -> (element #2=w598:string, element #3=w596:string)  [unwired: 3 in, 1 out]
          n153 = Equal?(x=w599, y=w598) -> (x = y?=w595:bool)
          n154 = Equal?(x=w597, y=w596) -> (x = y?=w594:bool)
          n155 = Compound Arithmetic op=AND(w595, w594) -> (w592:bool)
        }
        n156 = case shown="거짓" w570 {
          tunnel: w569 -> [_ w591]
          tunnel: [w577 w591] -> w568
          tunnel: w567 -> [w582 _]
          tunnel: w566 -> [w581 _]
          tunnel: w565 -> [w580 _]
          frame False {
            n157 = for {
              tunnel: w582 -> [w584] mode=indexing
              tunnel: w581 -> [w590]
              tunnel: w580 -> [w588]
              tunnel: [w584] -> w578
              tunnel: [w583] -> w579
              stop <- w583 stop-if-true
              n158 = Index Array(array=w584) -> (element #2=w589:string, element #3=w587:string)  [unwired: 3 in, 1 out]
              n159 = Equal?(x=w590, y=w589) -> (x = y?=w586:bool)
              n160 = Equal?(x=w588, y=w587) -> (x = y?=w585:bool)
              n161 = Compound Arithmetic op=AND(w586, w585) -> (w583:bool)
            }
            n162 = Select(t=w578, s=w579, f=string[] ["조합없음", "", "", "조합없음", "", "", "", "", "", "", "", "", "", "", "", "", "", "", "", "조합없음"]) -> (s? t:f=w577:string[])
          }
          frame True {
          }
        }
      }
      n163 = for {
        tunnel: w551 -> [w611] mode=indexing
        tunnel: [w610] -> w528 mode=indexing
        n164 = Index Array(array=w611, index #1=2 ("인덱스"), index #5=15 ("인덱스"), index #7=19 ("인덱스")) -> (element #1=w600:string, element #2=w603:string, element #3=w602:string, element #4=w614:string, element #5=w608:string, element #6=w607:string, element #7=w605:string, element #9=w604:string)  [unwired: 6 in, 1 out]
        n165 = Format Into String(format string="%s %s-%s" ("포맷 문자열"), w603, w602, w614) -> (resulting string=w612:string)  [unwired: 2 in, 1 out]
        n166 = Build Array(w612, w603, w602, w608, w607, w605, w604, w600) -> (w610:string[])
      }
      n167 = Delete From Array(array=w548, length=w538, index (col)=w539) -> (deleted portion=w531:string[][], array with subset deleted=w540:string[][])  [unwired: 1 in]
      n168 = call "Variables Data IO.vi"("Select"=Cmd_Var_Data_IO."Resolution", "error in"=w518, "Func_ext"=w547) -> ("error out"=w536:errorcluster, "Data Out"=w545:string[][], "Func_ext Out"=w525:string)  [unwired: 6 in]
      n169 = Delete From Array(array=w540, length=w538, index (col)=w539) -> (deleted portion=w529:string[][])  [unwired: 1 in, 1 out]
      n170 = Index Array(array=w545, index (row)=0 ("인덱스 (행)"), index (col)=2 ("비활성화된 인덱스 (열)")) -> (element=w541:string)
      n171 = case shown="\"Force_3_1\"" w525 {
        tunnel: ["Push" ("방향") "Pull" ("방향")] -> w532
        tunnel: w531 -> [_ w563]
        tunnel: [w561 w563] -> w530
        tunnel: w529 -> [w561 _]
        frame Default {
        }
        frame "Force_3_1" {
        }
      }
      n172 = call "Calcu_Force Weight.vi"("기준기 데이터"=w528, "방향"=w532, "분해능"=w541, "Condition"=w542, "분동조합"=w530) -> ("Condition Out"=w527:string[][], "사용기준추"=w535:string[][], "기준추 데이터"=w526:string[][])  [unwired: 3 in, 1 out]
      n173 = call "Variables Data IO.vi"("Write blank data ?(F)"=TRUE ("Write blank data ?(T)"), "Select"=Cmd_Var_Data_IO."STD2", "error in"=w536, "Data In"=w535, "Func_ext"=w525) -> ("error out"=w533:errorcluster)  [unwired: 4 in, 2 out]
    }
    frame "Frequency Meter" {
      n174 = case shown="\"Frequency Meter\", 기본" w618 {
        tunnel: ["Frequency Source"] -> w622
        tunnel: ["kHz" ("환산단위")] -> w621
        frame "Frequency Meter", Default {
        }
      }
      n175 = call-poly "Data Classification.vi"("인덱스"=2, "DATA 입력"=w629, "검색 문자열"=w622) -> ("DATA 출력"=w624:string[][])  [unwired: 4 in, 4 out]
      n176 = for {
        tunnel: w624 -> [w710] mode=indexing
        tunnel: [w705] -> w623 mode=indexing
        tunnel: w621 -> [w700]
        n177 = Index Array(array=w710, index #1=13 ("인덱스")) -> (element #1=w711:string, element #2=w709:string, element #3=w707:string, element #4=w708:string)  [unwired: 3 in]
        n178 = call "Unit Conversion.vi"("환산단위"=w700, "입력단위"=w708, "입력값"=w711) -> ("환산값 (string)"=w704:string)  [unwired: 3 in, 5 out]
        n179 = call "Unit Conversion.vi"("환산단위"=w700, "입력단위"=w708, "입력값"=w709) -> ("환산값 (string)"=w703:string)  [unwired: 3 in, 5 out]
        n180 = call "Unit Conversion.vi"("환산단위"=w700, "입력단위"=w708, "입력값"=w707) -> ("환산단위"=w701:string, "환산값 (string)"=w702:string)  [unwired: 3 in, 4 out]
        n181 = Replace Array Subset(array=w710, new element #1=w704, index #1=13 ("인덱스"), new element #2=w703, new element #3=w702, new element #4=w701) -> (w705:string[])  [unwired: 3 in]
      }
      n182 = call-poly "Data Sorting.vi"("기준열"=u16 13, "error in (no error)"=w628, "Data in"=w623) -> ("error out"=w626:errorcluster, "Data out"=w620:string[][])  [unwired: 7 in]
      n183 = for {
        tunnel: w620 -> [w653]
        tunnel: w627 -> [w652] mode=indexing
        tunnel: [w646] -> w619 mode=indexing
        w643 = 24 ("인덱스")
        w644 = 21 ("인덱스")
        w645 = 13 ("인덱스")
        n184 = Index Array(array=w652) -> (element #2=w649:string, element #3=w651:string)  [unwired: 3 in, 1 out]
        n185 = Fract/Exp String To Number(string=w649) -> (number=w650:dbl)  [unwired: 3 in, 1 out]
        n186 = for {
          tunnel: w653 -> [w666] mode=indexing
          tunnel: w651 -> [w654]
          tunnel: [w666] -> w647
          tunnel: w650 -> [w682]
          tunnel: w645 -> [w665]
          tunnel: w644 -> [w669]
          tunnel: w643 -> [w668]
          tunnel: [w667] -> w648
          tunnel: [w664] -> w642
          tunnel: [w663] -> w641
          tunnel: [w662] -> w640
          tunnel: [w661] -> w639
          tunnel: [w660] -> w638
          tunnel: [w659] -> w637
          tunnel: [w658] -> w636
          tunnel: [w657] -> w635
          tunnel: [w656] -> w634
          tunnel: [w655] -> w633
          stop <- w667 stop-if-true
          n187 = Index Array(array=w666, index #1=w665, index #8=w669, index #9=w668) -> (element #1=w684:string, element #2=w681:string, element #3=w680:string, element #4=w679:string, element #5=w678:string, element #6=w677:string, element #7=w676:string, element #8=w675:string, element #9=w674:string, element #10=w673:string, element #11=w671:string, element #12=w670:string)  [unwired: 9 in]
          n188 = call "Unit Conversion.vi"("환산단위"=w654, "입력단위"=w679, "입력값"=w684) -> ("환산단위"=w661:string, "환산값 (DBL)"=w683:dbl, "환산값 (string)"=w664:string)  [unwired: 3 in, 3 out]
          n189 = call "Unit Conversion.vi"("환산단위"=w654, "입력단위"=w679, "입력값"=w681) -> ("환산값 (string)"=w663:string)  [unwired: 3 in, 5 out]
          n190 = call "Unit Conversion.vi"("환산단위"=w654, "입력단위"=w679, "입력값"=w680) -> ("환산값 (string)"=w662:string)  [unwired: 3 in, 5 out]
          n191 = call "Unit Conversion.vi"("환산단위"=w654, "입력단위"=w677, "입력값"=w678) -> ("환산값 (string)"=w660:string)  [unwired: 3 in, 5 out]
          n192 = call "Unit Conversion.vi"("환산단위"=w654, "입력단위"=w675, "입력값"=w676) -> ("환산값 (string)"=w659:string)  [unwired: 3 in, 5 out]
          n193 = call "Unit Conversion.vi"("환산단위"="실수", "입력단위"=w673, "입력값"=w674) -> ("환산단위"=w657:string, "환산값 (string)"=w658:string)  [unwired: 3 in, 4 out]
          n194 = call "Unit Conversion.vi"("환산단위"=w654, "입력단위"=w670, "입력값"=w671) -> ("환산단위"=w655:string, "환산값 (string)"=w656:string)  [unwired: 3 in, 4 out]
          n195 = Greater Or Equal?(x=w683, y=w682) -> (x >= y?=w667:bool)
        }
        n196 = case shown="참" w648 {
          tunnel: w647 -> [_ w699]
          tunnel: [_ w698] -> w646
          tunnel: w645 -> [_ w697]
          tunnel: w642 -> [_ w696]
          tunnel: w641 -> [_ w695]
          tunnel: w640 -> [_ w694]
          tunnel: w639 -> [_ w691]
          tunnel: w638 -> [_ w693]
          tunnel: w637 -> [_ w692]
          tunnel: w636 -> [_ w688]
          tunnel: w644 -> [_ w690]
          tunnel: w635 -> [_ w687]
          tunnel: w643 -> [_ w689]
          tunnel: w634 -> [_ w686]
          tunnel: w633 -> [_ w685]
          frame False {
          }
          frame True {
            n197 = Replace Array Subset(array=w699, new element #1=w696, index #1=w697, new element #2=w695, new element #3=w694, new element #4=w691, new element #5=w693, new element #6=w691, new element #7=w692, new element #8=w691, index #8=w690, new element #9=w688, index #9=w689, new element #10=w687, new element #11=w686, new element #12=w685) -> (w698:string[])  [unwired: 9 in]
          }
        }
      }
    }
    frame "Mass_1_1", "Mass_1_2", "Mass_1_3" {
      w735 = TRUE ("Write blank data ?(T)")
      n198 = call-poly "Data Classification.vi"("인덱스"=2, "DATA 입력"=w754, "검색 문자열"="Weight") -> ("DATA 출력"=w751:string[][])  [unwired: 4 in, 4 out]
      n199 = call-poly "Data Sorting.vi"("기준열"=u16 3, "Data in"=w751) -> ("Data out"=w728:string[][])  [unwired: 8 in, 1 out]
      n200 = call "Create File Path.vi"("파일타입"=Cmd_File_Type."CSV", "항목"=Cmd_File_path."데이터파일경로", "에러 입력"=w718, "문자열 in"="Balance Cal Weight Set" ("delimiter (\\t)")) -> ("error out"=w716:errorcluster, "파일경로"=w717:path)  [unwired: 4 in, 2 out]
      n201 = call-poly "Data Classification.vi"("인덱스"=4, "대체 문자열"="20 kg" ("검색 문자열"), "DATA 입력"=w728, "검색 문자열"="20 kg(1)") -> ("DATA 출력"=w729:string[][])  [unwired: 3 in, 4 out]
      n202 = call-poly <vilib>:"Read Delimited Spreadsheet.vi"("file path (dialog if empty)"=w717, "delimiter (\\t)"="," ("delimiter (\\t)")) -> ("all rows"=w715:string[][])  [unwired: 8 in, 5 out]
      n203 = Index Array(array=w729) -> (element=w727:string[])  [unwired: 2 in]
      n204 = Delete From Array(array=w715, index (row)=0 ("인덱스 (행)")) -> (array with subset deleted=w714:string[][])  [unwired: 2 in, 1 out]
      n205 = Insert Into Array(array=w728, new element=w727) -> (w723:string[][])  [unwired: 2 in]
      n206 = for {
        tunnel: [w781] -> w733 mode=indexing
        tunnel: [w776] -> w746 mode=concatenating
        tunnel: w723 -> [w785]
        tunnel: [w780] -> w724 mode=indexing
        tunnel: [w782] -> w732 mode=indexing
        tunnel: [w770] -> w734
        tunnel: w714 -> [w772]
        tunnel: w713 -> [w774] mode=indexing
        n207 = Index Array(array=w774) -> (element #1=w773:string, element #2=w770:string)  [unwired: 2 in]
        n208 = case shown="기본" w770 {
          selector: w770 -> [_ w787]
          tunnel: w772 -> [w786 w789]
          tunnel: [w786 w788] -> w771
          frame "g" {
          }
          frame Default {
            n209 = for {
              tunnel: w789 -> [w791] mode=indexing
              tunnel: [w795] -> w788 mode=indexing
              tunnel: w787 -> [w790]
              n210 = Index Array(array=w791) -> (element=w794:string)  [unwired: 1 in]
              n211 = call "Unit Conversion.vi"("환산단위"=w790, "입력단위"="g", "입력값"=w794) -> ("환산값 (string)"=w792:string)  [unwired: 3 in, 5 out]
              n212 = Replace Array Subset(array=w791, new element=w792) -> (w795:string[])  [unwired: 1 in]
            }
          }
        }
        n213 = call-poly "Data Classification.vi"("인덱스"=0, "DATA 입력"=w771, "검색 문자열"=w773) -> ("DATA 출력"=w779:string[][])  [unwired: 4 in, 4 out]
        n214 = Delete From Array(array=w779, index (col)=0 ("인덱스")) -> (array with subset deleted=w777:string[][])  [unwired: 2 in, 1 out]
        n215 = for {
          tunnel: w785 -> [w804]
          tunnel: [w797] -> w784
          tunnel: [w802] -> w783
          tunnel: [w801] -> w781
          tunnel: [w800] -> w780
          tunnel: w770 -> [w799]
          tunnel: w773 -> [w798]
          tunnel: w777 -> [w796] mode=indexing
          tunnel: [w796] -> w776
          stop <- w797 continue-if-true
          n216 = case shown="기본" w798 {
            tunnel: w804 -> [w811 _]
            tunnel: [w810 w834] -> w800
            tunnel: [w809 w834] -> w802
            tunnel: w796 -> [w808 _]
            tunnel: w796 -> [w807 _]
            tunnel: [w807 w834] -> w801
            tunnel: [w806 _] -> w803
            tunnel: w799 -> [w805 _]
            frame Default {
              n217 = for {
                tunnel: w808 -> [w813] mode=indexing
                tunnel: w811 -> [w817]
                tunnel: [w816] -> w810 mode=indexing
                tunnel: [w815] -> w809 mode=indexing
                tunnel: [w814] -> w806 mode=indexing
                tunnel: w805 -> [w812]
                n218 = case shown="기본" w813 {
                  selector: w813 -> [_ w829]
                  tunnel: w817 -> [_ w831]
                  tunnel: [_ w827] -> w816
                  tunnel: [_ w820] -> w815
                  tunnel: [_ w828] -> w814
                  tunnel: w812 -> [_ w819]
                  frame "" {
                  }
                  frame Default {
                    n219 = Index Array(array=w831, index (col)=4 ("비활성화된 인덱스 (열)")) -> (element=w832:string[])  [unwired: 1 in]
                    n220 = Search 1D Array(1D array=w832, element=w829) -> (index of element=w825:i32)  [unwired: 1 in]
                    n221 = Index Array(array=w831, index (row) #1=w825, index (col) #1=15 ("비활성화된 인덱스 (열)"), index (row) #2=w825, index (col) #2=16 ("비활성화된 인덱스 (열)"), index (row) #3=w825, index (col) #3=24 ("비활성화된 인덱스 (열)")) -> (element #1=w823:string, element #2=w818:string, element #3=w820:string)
                    n222 = Less Than 0?(x=w825) -> (x < 0?=w828:bool)
                    n223 = call "Unit Conversion.vi"("환산단위"=w819, "입력단위"=w818, "입력값"=w823) -> ("환산값 (string)"=w822:string)  [unwired: 3 in, 5 out]
                    n224 = Select(t="에러", s=w828, f=w822) -> (s? t:f=w827:string)
                  }
                }
              }
            }
            frame "0" {
              w834 = string[] ["0"] ("t")
            }
          }
          n225 = Or Array Elements(Boolean array=w803) -> (logical OR=w797:bool)
        }
        n226 = case shown="참" w784 {
          tunnel: w783 -> [w835 _]
          tunnel: [w835 _] -> w782
          frame False {
          }
          frame True {
          }
        }
      }
      n227 = call-poly "Array Deduplication.vi"("error in (no error)"=w716, "배열 in"=w746) -> ("error out"=w742:errorcluster, "배열 out"=w745:string[])  [unwired: 8 in]
      n228 = for {
        tunnel: w745 -> [w769] mode=indexing
        tunnel: w723 -> [w768]
        tunnel: [w760] -> w736 mode=indexing
        tunnel: w734 -> [w757]
        n229 = Index Array(array=w768, index (col)=4 ("비활성화된 인덱스 (열)")) -> (element=w766:string[])  [unwired: 1 in]
        n230 = Search 1D Array(1D array=w766, element=w769) -> (index of element=w763:i32)  [unwired: 1 in]
        n231 = Index Array(array=w768, index (row) #1=w763, index (col) #1=4 ("비활성화된 인덱스 (열)"), index (row) #2=w763, index (col) #2=19 ("인덱스 (열)"), index (row) #3=w763, index (col) #3=21 ("비활성화된 인덱스 (열)")) -> (element #1=w761:string, element #2=w759:string, element #3=w758:string)
        n232 = call "Unit Conversion.vi"("환산단위"=w757, "입력단위"=w758, "입력값"=w759) -> ("환산단위"=w755:string, "환산값 (string)"=w756:string)  [unwired: 3 in, 4 out]
        n233 = Build Array(w761, w756, w755) -> (w760:string[])
      }
      n234 = call "Variables Data IO.vi"("Write blank data ?(F)"=w735, "Select"=Cmd_Var_Data_IO."STD2", "error in"=w742, "Data In"=w724, "Func_ext"=w722) -> ("error out"=w741:errorcluster, "Func_ext Out"=w743:string)  [unwired: 4 in, 1 out]
      n235 = call "Variables Data IO.vi"("Write blank data ?(F)"=w735, "Select"=Cmd_Var_Data_IO."STD3", "error in"=w741, "Data In"=w732, "Func_ext"=w743) -> ("error out"=w739:errorcluster, "Func_ext Out"=w737:string)  [unwired: 4 in, 1 out]
      n236 = Insert Into Array(array=w733, new element #1=w724, new element #2=w732) -> (w731:string[][])  [unwired: 2 in]
      n237 = call "Variables Data IO.vi"("Write blank data ?(F)"=w735, "Select"=Cmd_Var_Data_IO."STD4", "error in"=w739, "Data In"=w736, "Func_ext"=w737) -> ("error out"=w738:errorcluster)  [unwired: 4 in, 2 out]
    }
    frame "Mass_2_1", "Mass_2_2" {
      w846 = TRUE ("Write blank data ?(T)")
      n238 = call-poly "Data Classification.vi"("인덱스"=2, "DATA 입력"=w856, "검색 문자열"="Weight") -> ("DATA 출력"=w837:string[][])  [unwired: 4 in, 4 out]
      n239 = call-poly "Data Classification.vi"("인덱스"=2, "DATA 입력"=w856, "검색 문자열"="Electric Balance") -> ("DATA 출력"=w842:string[][])  [unwired: 4 in, 4 out]
      n240 = call-poly "Data Sorting.vi"("기준열"=u16 13, "Data in"=w842) -> ("Data out"=w838:string[][])  [unwired: 8 in, 1 out]
      n241 = for {
        tunnel: w847 -> [w922] mode=indexing
        tunnel: w837 -> [w863]
        tunnel: [w858] -> w836 mode=indexing
        tunnel: w838 -> [w917]
        tunnel: [w916] -> w854 mode=indexing
        tunnel: [w910] -> w849 mode=indexing
        tunnel: w845 -> [w886]
        w906 = "mg" ("환산단위")
        w907 = "g" ("환산단위")
        w893 = 24 ("비활성화된 인덱스 (열)")
        w888 = 21 ("비활성화된 인덱스 (열)")
        w891 = 19 ("비활성화된 인덱스 (열)")
        w896 = 15 ("비활성화된 인덱스 (열)")
        n242 = case shown="기본" w886 {
          tunnel: w922 -> [w944 w950]
          tunnel: [w935 w949] -> w918
          tunnel: [w938 w947] -> w885
          tunnel: [w936 w947] -> w884
          tunnel: [w936 w947] -> w872
          tunnel: [w935 w949] -> w870
          tunnel: ["추" ("문자열") w945] -> w864
          frame "Mass_2_2" {
            n243 = Index Array(array=w944, index #1=3 ("인덱스")) -> (element #1=w937:string, element #2=w936:string, element #3=w935:string)  [unwired: 2 in]
            n244 = Fract/Exp String To Number(string=w937) -> (number=w941:dbl)  [unwired: 3 in, 1 out]
            n245 = Fract/Exp String To Number(string=w936) -> (number=w942:dbl)  [unwired: 3 in, 1 out]
            n246 = Max & Min(x=w941, y=w942) -> (max(x,y)=w940:dbl)  [unwired: 1 out]
            n247 = Format Into String(format string="%#f" ("포맷 문자열"), w940) -> (resulting string=w938:string)  [unwired: 2 in, 1 out]
          }
          frame Default {
            n248 = Index Array(array=w950, index #1=4 ("인덱스"), index #3=1 ("인덱스")) -> (element #1=w947:string, element #2=w949:string, element #3=w945:string)  [unwired: 1 in]
          }
        }
        n249 = case shown="기본" w864 {
          tunnel: w863 -> [w926 w927 w929]
          tunnel: [w924 w927 w928] -> w862
          frame "F1" {
            n250 = call-poly "Data Classification.vi"("인덱스"=5, "DATA 입력"=w926, "검색 문자열"="E2") -> ("DATA 출력"=w924:string[][])  [unwired: 4 in, 4 out]
          }
          frame "추" {
          }
          frame Default {
            n251 = call-poly "Data Classification.vi"("인덱스"=5, "DATA 입력"=w929, "검색 문자열"="F1") -> ("DATA 출력"=w930:string[][])  [unwired: 4 in, 4 out]
            n252 = Empty Array?(array=w930) -> (empty?=w931:bool)
            n253 = Select(t=w929, s=w931, f=w930) -> (s? t:f=w928:string[][])
          }
        }
        n254 = Fract/Exp String To Number(string=w884) -> (number=w874:dbl)  [unwired: 3 in, 1 out]
        n255 = Equal?(x=w874, y=0.5) -> (x = y?=w876:bool)
        n256 = Equal?(x=w874, y=0.05) -> (x = y?=w882:bool)
        n257 = Select(t="1 g" ("원소"), s=w876, f="500 mg" ("원소")) -> (s? t:f=w873:string)
        n258 = Select(t="100 mg" ("원소"), s=w882, f="50 mg" ("원소")) -> (s? t:f=w879:string)
        n259 = for {
          tunnel: w885 -> [w975]
          tunnel: w918 -> [w955]
          tunnel: w917 -> [w968] mode=indexing
          tunnel: 16 ("비활성화된 인덱스 (열)") -> [w971]
          tunnel: 13 ("인덱스 (열)") -> [w970]
          tunnel: [w960] -> w916
          tunnel: 24 ("인덱스 (열)") -> [w967]
          tunnel: [w963] -> w914
          tunnel: 1 ("인덱스 (열)") -> [w962]
          tunnel: 34 ("인덱스 (열)") -> [w959]
          tunnel: [w957] -> w910
          tunnel: w879 -> [w952]
          tunnel: w873 -> [w951]
          stop <- w972 stop-if-true
          n260 = Index Array(array=w968, index #1=w971, index #2=w970, index #3=w967, index #4=w962, index #5=w959) -> (element #1=w956:string, element #2=w969:string, element #3=w954:string, element #4=w961:string, element #5=w958:string)
          n261 = Fract/Exp String To Number(string=w954) -> (number=w966:dbl)  [unwired: 3 in, 1 out]
          n262 = call "Unit Conversion.vi"("환산단위"=w956, "입력단위"=w955, "입력값"=w975) -> ("환산값 (DBL)"=w973:dbl)  [unwired: 3 in, 5 out]
          n263 = Fract/Exp String To Number(string=w969) -> (number=w974:dbl)  [unwired: 3 in, 1 out]
          n264 = Build Array(w961, w954, w958) -> (w960:string[])
          n265 = Build Array(w954, "g" ("입력단위")) -> (w957:string[])
          n266 = Greater Or Equal?(x=w966, y=0.01) -> (x >= y?=w964:bool)
          n267 = Less Or Equal?(x=w973, y=w974) -> (x <= y?=w972:bool)
          n268 = Select(t=w951, s=w964, f=w952) -> (s? t:f=w963:string)
        }
        n269 = call "Unit Conversion.vi"("환산단위"="g", "입력단위"=w870, "입력값"=w872) -> ("환산값 (string)"=w871:string)  [unwired: 3 in, 5 out]
        n270 = Index Array(array=w862, index (col) #1=13 ("비활성화된 인덱스 (열)"), index (col) #2=4 ("비활성화된 인덱스 (열)")) -> (element #1=w867:string[], element #2=w865:string[])  [unwired: 2 in]
        n271 = Search 1D Array(1D array=w867, element=w871) -> (index of element=w861:i32)  [unwired: 1 in]
        n272 = Search 1D Array(1D array=w865, element=w914) -> (index of element=w889:i32)  [unwired: 1 in]
        n273 = Index Array(array=w862, index (row) #1=w861, index (col) #1=3 ("비활성화된 인덱스 (열)"), index (row) #4=w861, index (col) #4=w896, index (row) #6=w861, index (col) #6=w893, index (row) #7=w861, index (col) #7=w891, index (row) #8=w861, index (col) #8=w888, index (row) #9=w889, index (col) #9=w896, index (row) #11=w889, index (col) #11=w893, index (row) #12=w889, index (col) #12=w891, index (row) #13=w889, index (col) #13=w888) -> (element #1=w904:string, element #2=w903:string, element #3=w902:string, element #4=w901:string, element #5=w900:string, element #6=w899:string, element #7=w898:string, element #8=w897:string, element #9=w895:string, element #10=w894:string, element #11=w892:string, element #12=w890:string, element #13=w887:string)  [unwired: 8 in]
        n274 = call "Unit Conversion.vi"("환산단위"=w907, "입력단위"=w900, "입력값"=w901) -> ("환산값 (string)"=w915:string)  [unwired: 3 in, 5 out]
        n275 = call "Unit Conversion.vi"("환산단위"=w906, "입력단위"=w897, "입력값"=w898) -> ("환산값 (string)"=w909:string)  [unwired: 3 in, 5 out]
        n276 = call "Unit Conversion.vi"("환산단위"=w907, "입력단위"=w894, "입력값"=w895) -> ("환산값 (string)"=w913:string)  [unwired: 3 in, 5 out]
        n277 = call "Unit Conversion.vi"("환산단위"=w906, "입력단위"=w887, "입력값"=w890) -> ("환산값 (string)"=w908:string)  [unwired: 3 in, 5 out]
        n278 = Less Than 0?(x=w861) -> (x < 0?=w860:bool)
        n279 = Build Array(w904, w903, w902, w915, w899, w909, w914, w913, w892, w908) -> (w859:string[])
        n280 = Select(t=string[] [], s=w860, f=w859) -> (s? t:f=w858:string[])
      }
      n281 = call "Variables Data IO.vi"("Write blank data ?(F)"=w846, "Select"=Cmd_Var_Data_IO."Resolution", "error in"=w852, "Data In"=w849, "Func_ext"=w845) -> ("error out"=w851:errorcluster, "Func_ext Out"=w848:string)  [unwired: 4 in, 1 out]
      n282 = call "Variables Data IO.vi"("Write blank data ?(F)"=w846, "Select"=Cmd_Var_Data_IO."STD2", "error in"=w851, "Data In"=w854, "Func_ext"=w848) -> ("error out"=w853:errorcluster)  [unwired: 4 in, 2 out]
    }
    frame "Pressure_1", "Pressure_2", "Pressure_3" {
      n283 = case shown="\"20414-0\"" w981 {
        tunnel: [string[][] [] ("STD Data") w1008 w1190 w1290 w1431 w1620 w1763 w1840] -> w987
        tunnel: [string[][] [] ("Data Out") w1009 w1189 w1291 w1430 w1619 w1764 w1841] -> w980
        tunnel: w986 -> [w1005 w1011 w1188 w1293 w1448 w1635 w1766 w1843]
        tunnel: w985 -> [_ w1012 w1186 w1294 w1449 w1636 w1767 w1844]
        tunnel: [w1005 w1010 w1167 w1292 w1434 w1623 w1765 w1842] -> w984
        tunnel: w983 -> [_ w1013 w1156 w1295 w1427 w1616 w1768 w1845]
        tunnel: w982 -> [_ w1014 w1139 w1296 w1420 w1609 w1769 w1846]
        tunnel: w977 -> [_ _ _ _ _ _ _ _]
        tunnel: w976 -> [_ _ _ _ _ _ _ w1838]
        frame Default {
        }
        frame "20406-0" {
          w1022 = 1.0 ("하위 리미트")
          w1029 = TRUE ("Write blank data ?(T)")
          w1026 = u16 11 ("기준열")
          w1049 = 0 ("인덱스 (행)")
          n284 = for {
            tunnel: w1014 -> [w1076] mode=indexing
            tunnel: [w1074] -> w1017 mode=indexing
            tunnel: [w1073] -> w1015 mode=indexing
            n285 = Index Array(array=w1076) -> (element=w1078:string)  [unwired: 1 in]
            n286 = Search and Replace String(input string=w1078, search string="-" ("검색 문자열")) -> (result string=w1075:string, offset past replacement=w1073:i32)  [unwired: 6 in, 2 out]
            n287 = Replace Array Subset(array=w1076, new element=w1075) -> (w1074:string[])  [unwired: 1 in]
          }
          n288 = call "Variables Data IO.vi"("Select"=Cmd_Var_Data_IO."Resolution", "error in"=w1011, "Func_ext"=w1012) -> ("error out"=w1034:errorcluster, "Data Out"=w1056:string[][], "Func_ext Out"=w1031:string)  [unwired: 6 in]
          n289 = Index Array(array=w1017, index (col) #1=w1049, index (row) #2=w1049, index (col) #2=1 ("비활성화된 인덱스 (열)")) -> (element #1=w1048:string[], element #2=w1054:string)  [unwired: 1 in]
          n290 = for {
            tunnel: w1013 -> [w1113] mode=indexing
            shift-right: [w1120] -> w1053
            shift-left: string[][] [] -> [w1119]
            tunnel: w1054 -> [w1110]
            tunnel: [w1113] -> w1042 mode=indexing if=w1115
            n291 = Index Array(array=w1113, index #1=13 ("인덱스"), index #2=16 ("인덱스"), index #3=2 ("인덱스")) -> (element #1=w1112:string, element #2=w1111:string, element #3=w1114:string)
            n292 = Equal?(x=w1114, y="Pressure Balance(abs)") -> (x = y?=w1123:bool)
            n293 = Equal?(x=w1114, y="Pressure Calibrator(abs)") -> (x = y?=w1122:bool)
            n294 = Equal?(x=w1114, y="Dead Weight") -> (x = y?=w1115:bool)
            n295 = Or(x=w1123, y=w1122) -> (x .or. y?=w1121:bool)
            n296 = case shown="참" w1121 {
              tunnel: w1113 -> [_ w1132]
              tunnel: [w1127 w1137] -> w1120
              tunnel: w1119 -> [w1127 w1136]
              tunnel: w1112 -> [_ w1135]
              tunnel: w1111 -> [_ w1134]
              tunnel: w1110 -> [_ w1133]
              frame False {
              }
              frame True {
                n297 = call "Unit Conversion.vi"("환산단위"=w1133, "입력단위"=w1134, "입력값"=w1135) -> ("환산단위"=w1130:string, "환산값 (string)"=w1131:string)  [unwired: 3 in, 4 out]
                n298 = Replace Array Subset(array=w1132, new element #1=w1131, index #1=11 ("인덱스"), new element #2=w1130) -> (w1128:string[])  [unwired: 1 in]
                n299 = Build Array (concatenate)(w1136, w1128) -> (w1137:string[][])
              }
            }
          }
          n300 = Fract/Exp String To Number(string=w1048) -> (number=w1050:dbl[])  [unwired: 3 in, 1 out]
          n301 = for {
            tunnel: w1017 -> [w1090] mode=indexing
            tunnel: [w1086] -> w1025 mode=indexing
            n302 = Index Array(array=w1090) -> (element #1=w1089:string, element #2=w1088:string)  [unwired: 2 in]
            n303 = call "Unit Conversion.vi"("환산단위"="kPa abs.", "입력단위"=w1088, "입력값"=w1089) -> ("환산값 (DBL)"=w1086:dbl)  [unwired: 3 in, 5 out]
          }
          n304 = Absolute Value(x=w1050) -> (abs(x)=w1018:dbl[])
          n305 = Array Max & Min(array=w1018) -> (max value=w1027:dbl)  [unwired: 3 out]
          n306 = Absolute Value(x=w1025) -> (abs(x)=w1020:dbl[])
          n307 = call-poly "Data Sorting.vi"("기준열"=w1026, "Data in"=w1053) -> ("Data out"=w1043:string[][])  [unwired: 8 in, 1 out]
          n308 = To Long Integer(number=w1026) -> (32bit integer=w1052:i32)
          n309 = Array Max & Min(array=w1020) -> (max value=w1021:dbl)  [unwired: 3 out]
          n310 = Index Array(array=w1043, index (col)=w1052) -> (element=w1051:string[])  [unwired: 1 in]
          n311 = In Range and Coerce(upper limit=1000.0 ("상위 리미트"), x=w1021, lower limit=w1022) -> (In Range?=w1023:bool)  [unwired: 1 out]
          n312 = Fract/Exp String To Number(string=w1051) -> (number=w1044:dbl[])  [unwired: 3 in, 1 out]
          n313 = case shown="참" w1023 {
            tunnel: [w1079 "kPa abs."] -> w1019
            tunnel: w1022 -> [w1084 _]
            tunnel: w1021 -> [w1083 _]
            frame False {
              n314 = Less?(x=w1083, y=w1084) -> (x < y?=w1082:bool)
              n315 = Select(t="Pa abs.", s=w1082, f="MPa abs.") -> (s? t:f=w1079:string)
            }
            frame True {
            }
          }
          n316 = for {
            tunnel: w1027 -> [w1108]
            tunnel: w1043 -> [w1107] mode=indexing
            tunnel: w1044 -> [w1109] mode=indexing
            tunnel: [w1107] -> w1047 if=w1106
            stop <- w1106 stop-if-true
            n317 = Less Or Equal?(x=w1108, y=w1109) -> (x <= y?=w1106:bool)
          }
          n318 = Index Array(array=w1047, index=2 ("인덱스")) -> (element=w1045:string)
          n319 = case shown="\"Pressure Balance\"" w1045 {
            tunnel: [w1092 w1105] -> w1008
            tunnel: [w1091 w1104] -> w1016
            tunnel: w1056 -> [w1094 w1103]
            tunnel: w1017 -> [w1093 w1102]
            tunnel: w1047 -> [w1095 w1101]
            tunnel: w1042 -> [w1099 _]
            tunnel: [w1098 _] -> w1036
            tunnel: [w1097 _] -> w1037
            tunnel: [w1096 _] -> w1032
            tunnel: w1019 -> [_ w1100]
            frame "Pressure Balance" {
              n320 = call "Calcu_STD Pressure_PB.vi"("Dead Weight"=w1099, "Resolution"=w1094, "Cal STD"=w1095, "Condition"=w1093) -> ("Mass set"=w1097:string[][], "Uncertainty"=w1098:string[][], "Data Out"=w1091:string[][], "STD Data"=w1092:string[][], "Weight set"=w1096:string[][])  [unwired: 2 in, 1 out]
            }
            frame Default {
              # "Pre"
              n321 = call "Calcu_STD Pressure_PC.vi"("STD 단위"=w1100, "Resolution"=w1103, "Cal STD (+)"=w1101, "Condition"=w1102) -> ("Data Out"=w1104:string[][], "STD Data"=w1105:string[][])  [unwired: 5 in, 1 out]
            }
          }
          n322 = for {
            tunnel: w1016 -> [w1059] mode=indexing
            tunnel: w1015 -> [w1060] mode=indexing
            tunnel: [w1058] -> w1009 mode=indexing
            n323 = case shown="기본" w1060 {
              tunnel: w1059 -> [w1067 w1072]
              tunnel: [w1063 w1072] -> w1058
              frame Default {
                w1070 = "-" ("문자열")
                w1061 = 4 ("인덱스")
                w1062 = 1 ("인덱스")
                n324 = Index Array(array=w1067, index #1=w1062, index #3=w1061) -> (element #1=w1071:string, element #2=w1069:string, element #3=w1068:string)  [unwired: 1 in]
                n325 = Concatenate Strings(w1070, w1071) -> (w1066:string)
                n326 = Concatenate Strings(w1070, w1069) -> (w1065:string)
                n327 = Concatenate Strings(w1070, w1068) -> (w1064:string)
                n328 = Replace Array Subset(array=w1067, new element #1=w1066, index #1=w1062, new element #2=w1065, new element #3=w1064, index #3=w1061) -> (w1063:string[])  [unwired: 1 in]
              }
              frame -1 {
              }
            }
          }
          n329 = call "Variables Data IO.vi"("Write blank data ?(F)"=w1029, "Select"=Cmd_Var_Data_IO."Condition_Temp", "error in"=w1034, "Data In"=w1032, "Func_ext"=w1031) -> ("error out"=w1033:errorcluster, "Func_ext Out"=w1030:string)  [unwired: 4 in, 1 out]
          n330 = call "Variables Data IO.vi"("Write blank data ?(F)"=w1029, "Select"=Cmd_Var_Data_IO."STD2", "error in"=w1033, "Data In"=w1037, "Func_ext"=w1030) -> ("error out"=w1039:errorcluster, "Func_ext Out"=w1038:string)  [unwired: 4 in, 1 out]
          n331 = call "Variables Data IO.vi"("Write blank data ?(F)"=w1029, "Select"=Cmd_Var_Data_IO."STD3", "error in"=w1039, "Data In"=w1036, "Func_ext"=w1038) -> ("error out"=w1010:errorcluster)  [unwired: 4 in, 2 out]
        }
        frame "20408-0", "20411-1", "20411-4" {
          w1142 = 1.0 ("하위 리미트")
          w1157 = TRUE ("Write blank data ?(T)")
          w1146 = u16 11 ("기준열")
          w1178 = 0 ("인덱스 (행)")
          w1155 = string[][] []
          n332 = Index Array(array=w1139, index (col) #1=w1178, index (row) #2=w1178, index (col) #2=1 ("비활성화된 인덱스 (열)")) -> (element #1=w1177:string[], element #2=w1183:string)  [unwired: 1 in]
          n333 = for {
            tunnel: w1156 -> [w1250] mode=indexing
            shift-right: [w1261] -> w1182
            shift-left: w1155 -> [w1260]
            tunnel: w1183 -> [w1247]
            tunnel: [w1250] -> w1171 mode=indexing if=w1256
            shift-right: [w1252] -> w1152
            shift-left: w1155 -> [w1253]
            n334 = Index Array(array=w1250, index #1=13 ("인덱스"), index #2=16 ("인덱스"), index #3=2 ("인덱스")) -> (element #1=w1249:string, element #2=w1248:string, element #3=w1255:string)
            n335 = Equal?(x=w1255, y="Pressure Balance") -> (x = y?=w1264:bool)
            n336 = Equal?(x=w1255, y="Pressure Calibrator(+)") -> (x = y?=w1263:bool)
            n337 = Equal?(x=w1255, y="Pressure Calibrator(-)") -> (x = y?=w1251:bool)
            n338 = Equal?(x=w1255, y="Dead Weight") -> (x = y?=w1256:bool)
            n339 = Or(x=w1264, y=w1263) -> (x .or. y?=w1262:bool)
            n340 = case shown="참" w1262 {
              tunnel: w1250 -> [_ w1284]
              tunnel: [w1279 w1289] -> w1261
              tunnel: w1260 -> [w1279 w1288]
              tunnel: w1249 -> [_ w1287]
              tunnel: w1248 -> [_ w1286]
              tunnel: w1247 -> [_ w1285]
              frame False {
              }
              frame True {
                n341 = call "Unit Conversion.vi"("환산단위"=w1285, "입력단위"=w1286, "입력값"=w1287) -> ("환산단위"=w1282:string, "환산값 (string)"=w1283:string)  [unwired: 3 in, 4 out]
                n342 = Replace Array Subset(array=w1284, new element #1=w1283, index #1=11 ("인덱스"), new element #2=w1282) -> (w1280:string[])  [unwired: 1 in]
                n343 = Build Array (concatenate)(w1288, w1280) -> (w1289:string[][])
              }
            }
            n344 = case shown="참" w1251 {
              tunnel: w1250 -> [_ w1274]
              tunnel: [w1268 w1269] -> w1252
              tunnel: w1253 -> [w1268 w1278]
              tunnel: w1249 -> [_ w1277]
              tunnel: w1248 -> [_ w1276]
              tunnel: w1247 -> [_ w1275]
              frame False {
              }
              frame True {
                n345 = call "Unit Conversion.vi"("환산단위"=w1275, "입력단위"=w1276, "입력값"=w1277) -> ("환산단위"=w1272:string, "환산값 (string)"=w1273:string)  [unwired: 3 in, 4 out]
                n346 = Replace Array Subset(array=w1274, new element #1=w1273, index #1=11 ("인덱스"), new element #2=w1272) -> (w1270:string[])  [unwired: 1 in]
                n347 = Build Array (concatenate)(w1278, w1270) -> (w1269:string[][])
              }
            }
          }
          n348 = for {
            tunnel: w1139 -> [w1202] mode=indexing
            tunnel: [w1198] -> w1145 mode=indexing
            n349 = Index Array(array=w1202) -> (element #1=w1201:string, element #2=w1200:string)  [unwired: 2 in]
            n350 = call "Unit Conversion.vi"("환산단위"="kPa", "입력단위"=w1200, "입력값"=w1201) -> ("환산값 (DBL)"=w1198:dbl)  [unwired: 3 in, 5 out]
          }
          n351 = call "Variables Data IO.vi"("Select"=Cmd_Var_Data_IO."Resolution", "error in"=w1188, "Func_ext"=w1186) -> ("error out"=w1162:errorcluster, "Data Out"=w1185:string[][], "Func_ext Out"=w1159:string)  [unwired: 6 in]
          n352 = Absolute Value(x=w1145) -> (abs(x)=w1140:dbl[])
          n353 = Array Max & Min(array=w1140) -> (max value=w1141:dbl)  [unwired: 3 out]
          n354 = Fract/Exp String To Number(string=w1177) -> (number=w1179:dbl[])  [unwired: 3 in, 1 out]
          n355 = In Range and Coerce(upper limit=1000.0 ("상위 리미트"), x=w1141, lower limit=w1142) -> (In Range?=w1143:bool)  [unwired: 1 out]
          n356 = Array Max & Min(array=w1179) -> (max value=w1151:dbl, min value=w1147:dbl)  [unwired: 2 out]
          n357 = case shown="거짓" w1143 {
            tunnel: [w1191 "kPa"] -> w1138
            tunnel: w1142 -> [w1196 _]
            tunnel: w1141 -> [w1195 _]
            frame False {
              n358 = Less?(x=w1195, y=w1196) -> (x < y?=w1194:bool)
              n359 = Select(t="Pa", s=w1194, f="MPa") -> (s? t:f=w1191:string)
            }
            frame True {
            }
          }
          n360 = call-poly "Data Sorting.vi"("기준열"=w1146, "Data in"=w1182) -> ("Data out"=w1172:string[][])  [unwired: 8 in, 1 out]
          n361 = call-poly "Data Sorting.vi"("기준열"=w1146, "Data in"=w1152) -> ("Data out"=w1149:string[][])  [unwired: 8 in, 1 out]
          n362 = To Long Integer(number=w1146) -> (32bit integer=w1181:i32)
          n363 = To Long Integer(number=w1146) -> (32bit integer=w1153:i32)
          n364 = Index Array(array=w1172, index (col)=w1181) -> (element=w1180:string[])  [unwired: 1 in]
          n365 = Index Array(array=w1149, index (col)=w1153) -> (element=w1154:string[])  [unwired: 1 in]
          n366 = Fract/Exp String To Number(string=w1180) -> (number=w1173:dbl[])  [unwired: 3 in, 1 out]
          n367 = Fract/Exp String To Number(string=w1154) -> (number=w1150:dbl[])  [unwired: 3 in, 1 out]
          n368 = for {
            tunnel: w1147 -> [w1205]
            tunnel: w1149 -> [w1204] mode=indexing
            tunnel: w1150 -> [w1206] mode=indexing
            tunnel: [w1204] -> w1148 if=w1203
            stop <- w1203 stop-if-true
            n369 = Greater Or Equal?(x=w1205, y=w1206) -> (x >= y?=w1203:bool)
          }
          n370 = for {
            tunnel: w1151 -> [w1245]
            tunnel: w1172 -> [w1244] mode=indexing
            tunnel: w1173 -> [w1246] mode=indexing
            tunnel: [w1244] -> w1176 if=w1243
            stop <- w1243 stop-if-true
            n371 = Less Or Equal?(x=w1245, y=w1246) -> (x <= y?=w1243:bool)
          }
          n372 = Index Array(array=w1176, index=2 ("인덱스")) -> (element=w1174:string)
          n373 = case shown="\"Pressure Balance\"" w1174 {
            tunnel: [w1208 w1242] -> w1190
            tunnel: [w1209 w1241] -> w1189
            tunnel: w1185 -> [w1216 w1240]
            tunnel: w1139 -> [w1215 w1239]
            tunnel: w1176 -> [w1218 w1238]
            tunnel: w1171 -> [w1222 _]
            tunnel: [w1221 _] -> w1164
            tunnel: [w1220 _] -> w1165
            tunnel: [w1219 _] -> w1160
            tunnel: w1148 -> [w1217 w1237]
            tunnel: w1138 -> [_ w1236]
            frame "Pressure Balance" {
              n374 = call "Calcu_STD Pressure_PC.vi"("STD 단위"="MPa", "Cal STD (-)"=w1217, "Resolution"=w1216, "Condition"=w1215) -> ("Data Out"=w1211:string[][], "STD Data"=w1213:string[][])  [unwired: 5 in, 1 out]
              n375 = call "Calcu_STD Pressure_PB.vi"("Dead Weight"=w1222, "Resolution"=w1216, "Cal STD"=w1218, "Condition"=w1215) -> ("Mass set"=w1220:string[][], "Uncertainty"=w1221:string[][], "Data Out"=w1210:string[][], "STD Data"=w1212:string[][], "Weight set"=w1219:string[][])  [unwired: 2 in, 1 out]
              n376 = Fract/Exp String To Number(string=w1215) -> (number=w1214:dbl[][])  [unwired: 3 in, 1 out]
              n377 = for {
                tunnel: w1214 -> [w1231] mode=indexing
                tunnel: w1213 -> [w1228] mode=indexing
                tunnel: w1212 -> [w1227] mode=indexing
                tunnel: w1211 -> [w1226] mode=indexing
                tunnel: w1210 -> [w1225] mode=indexing
                tunnel: [w1224] -> w1209 mode=indexing
                tunnel: [w1223] -> w1208 mode=indexing
                n378 = Index Array(array=w1231) -> (element=w1230:dbl)  [unwired: 1 in]
                n379 = Less Than 0?(x=w1230) -> (x < 0?=w1229:bool)
                n380 = case shown="거짓" w1229 {
                  tunnel: w1228 -> [_ w1235]
                  tunnel: w1227 -> [w1233 _]
                  tunnel: [w1233 w1235] -> w1223
                  tunnel: w1226 -> [_ w1234]
                  tunnel: [w1232 w1234] -> w1224
                  tunnel: w1225 -> [w1232 _]
                  frame False {
                  }
                  frame True {
                  }
                }
              }
            }
            frame Default {
              # "Pre"
              n381 = call "Calcu_STD Pressure_PC.vi"("STD 단위"=w1236, "Cal STD (-)"=w1237, "Resolution"=w1240, "Cal STD (+)"=w1238, "Condition"=w1239) -> ("Data Out"=w1241:string[][], "STD Data"=w1242:string[][])  [unwired: 4 in, 1 out]
            }
          }
          n382 = call "Variables Data IO.vi"("Write blank data ?(F)"=w1157, "Select"=Cmd_Var_Data_IO."Condition_Temp", "error in"=w1162, "Data In"=w1160, "Func_ext"=w1159) -> ("error out"=w1161:errorcluster, "Func_ext Out"=w1158:string)  [unwired: 4 in, 1 out]
          n383 = call "Variables Data IO.vi"("Write blank data ?(F)"=w1157, "Select"=Cmd_Var_Data_IO."STD2", "error in"=w1161, "Data In"=w1165, "Func_ext"=w1158) -> ("error out"=w1168:errorcluster, "Func_ext Out"=w1166:string)  [unwired: 4 in, 1 out]
          n384 = call "Variables Data IO.vi"("Write blank data ?(F)"=w1157, "Select"=Cmd_Var_Data_IO."STD3", "error in"=w1168, "Data In"=w1164, "Func_ext"=w1166) -> ("error out"=w1167:errorcluster)  [unwired: 4 in, 2 out]
        }
        frame "20409-0" {
          w1304 = 1.0 ("하위 리미트")
          w1311 = TRUE ("Write blank data ?(T)")
          w1308 = u16 11 ("기준열")
          w1331 = 0 ("인덱스 (행)")
          n385 = for {
            tunnel: w1296 -> [w1358] mode=indexing
            tunnel: [w1356] -> w1299 mode=indexing
            tunnel: [w1355] -> w1297 mode=indexing
            n386 = Index Array(array=w1358) -> (element=w1360:string)  [unwired: 1 in]
            n387 = Search and Replace String(input string=w1360, search string="-" ("검색 문자열")) -> (result string=w1357:string, offset past replacement=w1355:i32)  [unwired: 6 in, 2 out]
            n388 = Replace Array Subset(array=w1358, new element=w1357) -> (w1356:string[])  [unwired: 1 in]
          }
          n389 = call "Variables Data IO.vi"("Select"=Cmd_Var_Data_IO."Resolution", "error in"=w1293, "Func_ext"=w1294) -> ("error out"=w1316:errorcluster, "Data Out"=w1338:string[][], "Func_ext Out"=w1313:string)  [unwired: 6 in]
          n390 = Index Array(array=w1299, index (col) #1=w1331, index (row) #2=w1331, index (col) #2=1 ("비활성화된 인덱스 (열)")) -> (element #1=w1330:string[], element #2=w1336:string)  [unwired: 1 in]
          n391 = for {
            tunnel: w1295 -> [w1395] mode=indexing
            shift-right: [w1402] -> w1335
            shift-left: string[][] [] -> [w1401]
            tunnel: w1336 -> [w1392]
            tunnel: [w1395] -> w1324 mode=indexing if=w1397
            n392 = Index Array(array=w1395, index #1=13 ("인덱스"), index #2=16 ("인덱스"), index #3=2 ("인덱스")) -> (element #1=w1394:string, element #2=w1393:string, element #3=w1396:string)
            n393 = Equal?(x=w1396, y="Pressure Balance") -> (x = y?=w1405:bool)
            n394 = Equal?(x=w1396, y="Pressure Calibrator(+)") -> (x = y?=w1404:bool)
            n395 = Equal?(x=w1396, y="Dead Weight") -> (x = y?=w1397:bool)
            n396 = Or(x=w1405, y=w1404) -> (x .or. y?=w1403:bool)
            n397 = case shown="참" w1403 {
              tunnel: w1395 -> [_ w1414]
              tunnel: [w1409 w1419] -> w1402
              tunnel: w1401 -> [w1409 w1418]
              tunnel: w1394 -> [_ w1417]
              tunnel: w1393 -> [_ w1416]
              tunnel: w1392 -> [_ w1415]
              frame False {
              }
              frame True {
                n398 = call "Unit Conversion.vi"("환산단위"=w1415, "입력단위"=w1416, "입력값"=w1417) -> ("환산단위"=w1412:string, "환산값 (string)"=w1413:string)  [unwired: 3 in, 4 out]
                n399 = Replace Array Subset(array=w1414, new element #1=w1413, index #1=11 ("인덱스"), new element #2=w1412) -> (w1410:string[])  [unwired: 1 in]
                n400 = Build Array (concatenate)(w1418, w1410) -> (w1419:string[][])
              }
            }
          }
          n401 = Fract/Exp String To Number(string=w1330) -> (number=w1332:dbl[])  [unwired: 3 in, 1 out]
          n402 = Absolute Value(x=w1332) -> (abs(x)=w1300:dbl[])
          n403 = for {
            tunnel: w1299 -> [w1372] mode=indexing
            tunnel: [w1368] -> w1307 mode=indexing
            n404 = Index Array(array=w1372) -> (element #1=w1371:string, element #2=w1370:string)  [unwired: 2 in]
            n405 = call "Unit Conversion.vi"("환산단위"="kPa", "입력단위"=w1370, "입력값"=w1371) -> ("환산값 (DBL)"=w1368:dbl)  [unwired: 3 in, 5 out]
          }
          n406 = Array Max & Min(array=w1300) -> (max value=w1309:dbl)  [unwired: 3 out]
          n407 = Absolute Value(x=w1307) -> (abs(x)=w1302:dbl[])
          n408 = call-poly "Data Sorting.vi"("기준열"=w1308, "Data in"=w1335) -> ("Data out"=w1325:string[][])  [unwired: 8 in, 1 out]
          n409 = To Long Integer(number=w1308) -> (32bit integer=w1334:i32)
          n410 = Array Max & Min(array=w1302) -> (max value=w1303:dbl)  [unwired: 3 out]
          n411 = Index Array(array=w1325, index (col)=w1334) -> (element=w1333:string[])  [unwired: 1 in]
          n412 = In Range and Coerce(upper limit=1000.0 ("상위 리미트"), x=w1303, lower limit=w1304) -> (In Range?=w1305:bool)  [unwired: 1 out]
          n413 = Fract/Exp String To Number(string=w1333) -> (number=w1326:dbl[])  [unwired: 3 in, 1 out]
          n414 = case shown="거짓" w1305 {
            tunnel: [w1361 "kPa"] -> w1301
            tunnel: w1304 -> [w1366 _]
            tunnel: w1303 -> [w1365 _]
            frame False {
              n415 = Less?(x=w1365, y=w1366) -> (x < y?=w1364:bool)
              n416 = Select(t="Pa", s=w1364, f="MPa") -> (s? t:f=w1361:string)
            }
            frame True {
            }
          }
          n417 = for {
            tunnel: w1309 -> [w1390]
            tunnel: w1325 -> [w1389] mode=indexing
            tunnel: w1326 -> [w1391] mode=indexing
            tunnel: [w1389] -> w1329 if=w1388
            stop <- w1388 stop-if-true
            n418 = Less Or Equal?(x=w1390, y=w1391) -> (x <= y?=w1388:bool)
          }
          n419 = Index Array(array=w1329, index=2 ("인덱스")) -> (element=w1327:string)
          n420 = case shown="\"Pressure Balance\"" w1327 {
            tunnel: [w1374 w1387] -> w1290
            tunnel: [w1373 w1386] -> w1298
            tunnel: w1338 -> [w1376 w1385]
            tunnel: w1299 -> [w1375 w1384]
            tunnel: w1329 -> [w1377 w1383]
            tunnel: w1324 -> [w1381 _]
            tunnel: [w1380 _] -> w1318
            tunnel: [w1379 _] -> w1319
            tunnel: [w1378 _] -> w1314
            tunnel: w1301 -> [_ w1382]
            frame "Pressure Balance" {
              n421 = call "Calcu_STD Pressure_PB.vi"("Dead Weight"=w1381, "Resolution"=w1376, "Cal STD"=w1377, "Condition"=w1375) -> ("Mass set"=w1379:string[][], "Uncertainty"=w1380:string[][], "Data Out"=w1373:string[][], "STD Data"=w1374:string[][], "Weight set"=w1378:string[][])  [unwired: 2 in, 1 out]
            }
            frame Default {
              # "Pre"
              n422 = call "Calcu_STD Pressure_PC.vi"("STD 단위"=w1382, "Resolution"=w1385, "Cal STD (+)"=w1383, "Condition"=w1384) -> ("Data Out"=w1386:string[][], "STD Data"=w1387:string[][])  [unwired: 5 in, 1 out]
            }
          }
          n423 = for {
            tunnel: w1298 -> [w1341] mode=indexing
            tunnel: w1297 -> [w1342] mode=indexing
            tunnel: [w1340] -> w1291 mode=indexing
            n424 = case shown="기본" w1342 {
              tunnel: w1341 -> [w1349 w1354]
              tunnel: [w1345 w1354] -> w1340
              frame Default {
                w1352 = "-" ("문자열")
                w1343 = 4 ("인덱스")
                w1344 = 1 ("인덱스")
                n425 = Index Array(array=w1349, index #1=w1344, index #3=w1343) -> (element #1=w1353:string, element #2=w1351:string, element #3=w1350:string)  [unwired: 1 in]
                n426 = Concatenate Strings(w1352, w1353) -> (w1348:string)
                n427 = Concatenate Strings(w1352, w1351) -> (w1347:string)
                n428 = Concatenate Strings(w1352, w1350) -> (w1346:string)
                n429 = Replace Array Subset(array=w1349, new element #1=w1348, index #1=w1344, new element #2=w1347, new element #3=w1346, index #3=w1343) -> (w1345:string[])  [unwired: 1 in]
              }
              frame -1 {
              }
            }
          }
          n430 = call "Variables Data IO.vi"("Write blank data ?(F)"=w1311, "Select"=Cmd_Var_Data_IO."Condition_Temp", "error in"=w1316, "Data In"=w1314, "Func_ext"=w1313) -> ("error out"=w1315:errorcluster, "Func_ext Out"=w1312:string)  [unwired: 4 in, 1 out]
          n431 = call "Variables Data IO.vi"("Write blank data ?(F)"=w1311, "Select"=Cmd_Var_Data_IO."STD2", "error in"=w1315, "Data In"=w1319, "Func_ext"=w1312) -> ("error out"=w1321:errorcluster, "Func_ext Out"=w1320:string)  [unwired: 4 in, 1 out]
          n432 = call "Variables Data IO.vi"("Write blank data ?(F)"=w1311, "Select"=Cmd_Var_Data_IO."STD3", "error in"=w1321, "Data In"=w1318, "Func_ext"=w1320) -> ("error out"=w1292:errorcluster)  [unwired: 4 in, 2 out]
        }
        frame "20412-1" {
          w1454 = 1.0 ("하위 리미트")
          w1460 = TRUE ("Write blank data ?(T)")
          w1458 = u16 11 ("기준열")
          w1480 = 0 ("인덱스 (행)")
          n433 = Index Array(array=w1420, index (row)=0 ("인덱스 (행)"), index (col)=5 ("비활성화된 인덱스 (열)")) -> (element=w1443:string)
          n434 = case shown="\"mA\"" w1443 {
            tunnel: ["DC Voltage Meter" ("검색 문자열") "DC Voltage Meter" ("검색 문자열") "DC Current Meter" ("검색 문자열")] -> w1442
            tunnel: ["V" "mV" "mA"] -> w1438
            frame Default {
            }
            frame "mV/V" {
            }
            frame "mA" {
            }
          }
          n435 = Index Array(array=w1420, index (col) #1=w1480, index (row) #2=w1480, index (col) #2=1 ("비활성화된 인덱스 (열)")) -> (element #1=w1479:string[], element #2=w1485:string)  [unwired: 1 in]
          n436 = for {
            tunnel: w1427 -> [w1585] mode=indexing
            shift-right: [w1591] -> w1484
            shift-left: string[][] [] -> [w1590]
            tunnel: w1485 -> [w1582]
            tunnel: [w1585] -> w1473 mode=indexing if=w1586
            n437 = Index Array(array=w1585, index #1=13 ("인덱스"), index #2=16 ("인덱스"), index #3=2 ("인덱스")) -> (element #1=w1584:string, element #2=w1583:string, element #3=w1581:string)
            n438 = Equal?(x=w1581, y="Pressure Balance") -> (x = y?=w1594:bool)
            n439 = Equal?(x=w1581, y="Pressure Calibrator(+)") -> (x = y?=w1593:bool)
            n440 = Equal?(x=w1581, y="Dead Weight") -> (x = y?=w1586:bool)
            n441 = Or(x=w1594, y=w1593) -> (x .or. y?=w1592:bool)
            n442 = case shown="참" w1592 {
              tunnel: w1585 -> [_ w1603]
              tunnel: [w1598 w1608] -> w1591
              tunnel: w1590 -> [w1598 w1607]
              tunnel: w1584 -> [_ w1606]
              tunnel: w1583 -> [_ w1605]
              tunnel: w1582 -> [_ w1604]
              frame False {
              }
              frame True {
                n443 = call "Unit Conversion.vi"("환산단위"=w1604, "입력단위"=w1605, "입력값"=w1606) -> ("환산단위"=w1601:string, "환산값 (string)"=w1602:string)  [unwired: 3 in, 4 out]
                n444 = Replace Array Subset(array=w1603, new element #1=w1602, index #1=11 ("인덱스"), new element #2=w1601) -> (w1599:string[])  [unwired: 1 in]
                n445 = Build Array (concatenate)(w1607, w1599) -> (w1608:string[][])
              }
            }
          }
          n446 = call-poly "Data Classification.vi"("인덱스"=2, "DATA 입력"=w1427, "검색 문자열"="DC Power Supply") -> ("행크기"=w1425:i32)  [unwired: 4 in, 4 out]
          n447 = Less Or Equal To 0?(x=w1425) -> (x <= 0?=w1424:bool)
          n448 = call-poly "Data Classification.vi"("인덱스"=2, "DATA 입력"=w1427, "검색 문자열"=w1442) -> ("DATA 출력"=w1440:string[][])  [unwired: 4 in, 4 out]
          n449 = for {
            tunnel: w1420 -> [w1559] mode=indexing
            tunnel: [w1555] -> w1457 mode=indexing
            n450 = Index Array(array=w1559) -> (element #1=w1558:string, element #2=w1557:string)  [unwired: 2 in]
            n451 = call "Unit Conversion.vi"("환산단위"="kPa", "입력단위"=w1557, "입력값"=w1558) -> ("환산값 (DBL)"=w1555:dbl)  [unwired: 3 in, 5 out]
          }
          n452 = Fract/Exp String To Number(string=w1479) -> (number=w1481:dbl[])  [unwired: 3 in, 1 out]
          n453 = call "Variables Data IO.vi"("Select"=Cmd_Var_Data_IO."Resolution", "error in"=w1448, "Func_ext"=w1449) -> ("error out"=w1465:errorcluster, "Data Out"=w1487:string[][], "Func_ext Out"=w1462:string)  [unwired: 6 in]
          n454 = Absolute Value(x=w1481) -> (abs(x)=w1450:dbl[])
          n455 = for {
            tunnel: w1440 -> [w1537] mode=indexing
            tunnel: [w1536] -> w1439 mode=indexing
            tunnel: w1438 -> [w1541]
            n456 = Index Array(array=w1537, index #1=13 ("인덱스"), index #2=16 ("인덱스")) -> (element #1=w1539:string, element #2=w1532:string)
            n457 = call "Unit Conversion.vi"("환산단위"=w1541, "입력단위"=w1532, "입력값"=w1539) -> ("환산단위"=w1533:string, "환산값 (string)"=w1534:string)  [unwired: 3 in, 4 out]
            n458 = Replace Array Subset(array=w1537, new element #1=w1534, index #1=11 ("인덱스"), new element #2=w1533) -> (w1536:string[])  [unwired: 1 in]
          }
          n459 = Array Max & Min(array=w1450) -> (max value=w1459:dbl)  [unwired: 3 out]
          n460 = Absolute Value(x=w1457) -> (abs(x)=w1452:dbl[])
          n461 = call-poly "Data Sorting.vi"("기준열"=w1458, "Data in"=w1484) -> ("Data out"=w1474:string[][])  [unwired: 8 in, 1 out]
          n462 = To Long Integer(number=w1458) -> (32bit integer=w1483:i32)
          n463 = Array Max & Min(array=w1452) -> (max value=w1453:dbl)  [unwired: 3 out]
          n464 = Select(t="error" ("검색 문자열"), s=w1424, f="ok") -> (s? t:f=w1421:string)
          n465 = Index Array(array=w1474, index (col)=w1483) -> (element=w1482:string[])  [unwired: 1 in]
          n466 = In Range and Coerce(upper limit=1000.0 ("상위 리미트"), x=w1453, lower limit=w1454) -> (In Range?=w1455:bool)  [unwired: 1 out]
          n467 = Fract/Exp String To Number(string=w1482) -> (number=w1475:dbl[])  [unwired: 3 in, 1 out]
          n468 = case shown="거짓" w1455 {
            tunnel: [w1548 "kPa"] -> w1451
            tunnel: w1454 -> [w1553 _]
            tunnel: w1453 -> [w1552 _]
            frame False {
              n469 = Less?(x=w1552, y=w1553) -> (x < y?=w1551:bool)
              n470 = Select(t="Pa", s=w1551, f="MPa") -> (s? t:f=w1548:string)
            }
            frame True {
            }
          }
          n471 = for {
            tunnel: w1459 -> [w1579]
            tunnel: w1474 -> [w1578] mode=indexing
            tunnel: w1475 -> [w1580] mode=indexing
            tunnel: [w1578] -> w1478 if=w1577
            stop <- w1577 stop-if-true
            n472 = Less Or Equal?(x=w1579, y=w1580) -> (x <= y?=w1577:bool)
          }
          n473 = call-poly "Data Sorting.vi"("기준열"=u16 11, "Data in"=w1439) -> ("Data out"=w1432:string[][])  [unwired: 8 in, 1 out]
          n474 = Index Array(array=w1478, index=2 ("인덱스")) -> (element=w1476:string)
          n475 = case shown="\"Pressure Balance\"" w1476 {
            tunnel: [w1562 w1576] -> w1431
            tunnel: [w1561 w1575] -> w1430
            tunnel: w1487 -> [w1564 w1574]
            tunnel: w1420 -> [w1563 w1573]
            tunnel: w1478 -> [w1565 w1572]
            tunnel: w1473 -> [w1569 _]
            tunnel: [w1568 _] -> w1467
            tunnel: [w1567 _] -> w1468
            tunnel: [w1566 _] -> w1463
            tunnel: w1451 -> [_ w1571]
            tunnel: [w1560 w1570] -> w1429
            frame "Pressure Balance" {
              n476 = call "Calcu_STD Pressure_PB.vi"("Dead Weight"=w1569, "Resolution"=w1564, "Cal STD"=w1565, "Condition"=w1563) -> ("Mass set"=w1567:string[][], "Uncertainty"=w1568:string[][], "Data Out"=w1561:string[][], "STD Data"=w1562:string[][], "Weight set"=w1566:string[][], "배열"=w1560:dbl[])  [unwired: 2 in]
            }
            frame Default {
              # "Pre"
              n477 = call "Calcu_STD Pressure_PC.vi"("STD 단위"=w1571, "Resolution"=w1574, "Cal STD (+)"=w1572, "Condition"=w1573) -> ("Data Out"=w1575:string[][], "STD Data"=w1576:string[][], "배열"=w1570:dbl[])  [unwired: 5 in]
            }
          }
          n478 = for {
            tunnel: [w1492] -> w1437 mode=indexing
            tunnel: w1432 -> [w1491]
            tunnel: w1429 -> [w1490] mode=indexing
            tunnel: w1421 -> [w1489]
            n479 = for {
              tunnel: [w1524] -> w1492
              tunnel: w1491 -> [w1522] mode=indexing
              tunnel: w1490 -> [w1505]
              tunnel: w1489 -> [w1493]
              stop <- w1530 stop-if-true
              n480 = Index Array(array=w1522, index #1=11 ("비활성화된 인덱스 (열)"), index #2=1 ("인덱스"), index #3=13 ("인덱스"), index #4=15 ("인덱스"), index #8=19 ("인덱스"), index #9=21 ("인덱스"), index #10=12 ("인덱스"), index #11=24 ("인덱스")) -> (element #1=w1503:string, element #2=w1501:string, element #3=w1499:string, element #4=w1497:string, element #5=w1496:string, element #6=w1507:string, element #7=w1506:string, element #8=w1528:string, element #9=w1518:string, element #10=w1495:string, element #11=w1515:string, element #12=w1514:string, element #13=w1520:string, element #14=w1519:string)  [unwired: 6 in]
              n481 = Fract/Exp String To Number(string=w1503) -> (number=w1531:dbl)  [unwired: 3 in, 1 out]
              n482 = call "Unit Conversion.vi"("환산단위"=w1495, "입력단위"=w1496, "입력값"=w1499) -> ("환산값 (string)"=w1508:string)  [unwired: 3 in, 5 out]
              n483 = call "Unit Conversion.vi"("환산단위"=w1495, "입력단위"=w1496, "입력값"=w1497) -> ("환산값 (string)"=w1494:string)  [unwired: 3 in, 5 out]
              n484 = call "Unit Conversion.vi"("환산단위"=w1495, "입력단위"=w1506, "입력값"=w1507) -> ("환산단위"=w1510:string, "환산값 (string)"=w1509:string)  [unwired: 3 in, 4 out]
              n485 = call "Unit Conversion.vi"("환산단위"=w1495, "입력단위"=w1518, "입력값"=w1528) -> ("환산단위"=w1523:string, "환산값 (string)"=w1525:string)  [unwired: 3 in, 4 out]
              n486 = call "Unit Conversion.vi"("환산단위"="실수", "입력단위"=w1514, "입력값"=w1515) -> ("환산단위"=w1511:string, "환산값 (string)"=w1512:string)  [unwired: 3 in, 4 out]
              n487 = call "Unit Conversion.vi"("환산단위"=w1495, "입력단위"=w1519, "입력값"=w1520) -> ("환산단위"=w1516:string, "환산값 (string)"=w1517:string)  [unwired: 3 in, 4 out]
              n488 = Less?(x=w1505, y=w1531) -> (x < y?=w1530:bool)
              n489 = Build Array(w1501, w1508, w1494, w1509, w1510, w1525, w1523, w1512, w1511, w1517, w1516, w1493) -> (w1524:string[])
            }
          }
          n490 = call "Variables Data IO.vi"("Write blank data ?(F)"=w1460, "Select"=Cmd_Var_Data_IO."Condition_Temp", "error in"=w1465, "Data In"=w1463, "Func_ext"=w1462) -> ("error out"=w1464:errorcluster, "Func_ext Out"=w1461:string)  [unwired: 4 in, 1 out]
          n491 = call "Variables Data IO.vi"("Write blank data ?(F)"=w1460, "Select"=Cmd_Var_Data_IO."STD2", "error in"=w1464, "Data In"=w1468, "Func_ext"=w1461) -> ("error out"=w1470:errorcluster, "Func_ext Out"=w1469:string)  [unwired: 4 in, 1 out]
          n492 = call "Variables Data IO.vi"("Write blank data ?(F)"=w1460, "Select"=Cmd_Var_Data_IO."STD3", "error in"=w1470, "Data In"=w1467, "Func_ext"=w1469) -> ("error out"=w1436:errorcluster, "Func_ext Out"=w1435:string)  [unwired: 4 in, 1 out]
          n493 = call "Variables Data IO.vi"("Select"=Cmd_Var_Data_IO."STD4", "error in"=w1436, "Data In"=w1437, "Func_ext"=w1435) -> ("error out"=w1434:errorcluster)  [unwired: 5 in, 2 out]
        }
        frame "20412-2" {
          w1641 = 1.0 ("하위 리미트")
          w1645 = u16 11 ("기준열")
          w1653 = 0 ("인덱스 (행)")
          n494 = Index Array(array=w1609, index (row)=0 ("인덱스 (행)"), index (col)=5 ("비활성화된 인덱스 (열)")) -> (element=w1630:string)
          n495 = case shown="\"mA\"" w1630 {
            tunnel: ["DC Voltage Meter" ("검색 문자열") "DC Voltage Meter" ("검색 문자열") "DC Current Meter" ("검색 문자열")] -> w1629
            tunnel: ["V" "mV" "mA"] -> w1625
            frame Default {
            }
            frame "mV/V" {
            }
            frame "mA" {
            }
          }
          n496 = Index Array(array=w1609, index (col) #1=w1653, index (row) #2=w1653, index (col) #2=1 ("비활성화된 인덱스 (열)")) -> (element #1=w1652:string[], element #2=w1658:string)  [unwired: 1 in]
          n497 = for {
            tunnel: w1616 -> [w1741] mode=indexing
            shift-right: [w1745] -> w1657
            shift-left: string[][] [] -> [w1744]
            tunnel: w1658 -> [w1738]
            n498 = Index Array(array=w1741, index #1=13 ("인덱스"), index #2=16 ("인덱스"), index #3=2 ("인덱스")) -> (element #1=w1740:string, element #2=w1739:string, element #3=w1737:string)
            n499 = Equal?(x=w1737, y="Pressure Balance") -> (x = y?=w1748:bool)
            n500 = Equal?(x=w1737, y="Pressure Calibrator(abs)") -> (x = y?=w1747:bool)
            n501 = Or(x=w1748, y=w1747) -> (x .or. y?=w1746:bool)
            n502 = case shown="참" w1746 {
              tunnel: w1741 -> [_ w1757]
              tunnel: [w1752 w1762] -> w1745
              tunnel: w1744 -> [w1752 w1761]
              tunnel: w1740 -> [_ w1760]
              tunnel: w1739 -> [_ w1759]
              tunnel: w1738 -> [_ w1758]
              frame False {
              }
              frame True {
                n503 = call "Unit Conversion.vi"("환산단위"=w1758, "입력단위"=w1759, "입력값"=w1760) -> ("환산단위"=w1755:string, "환산값 (string)"=w1756:string)  [unwired: 3 in, 4 out]
                n504 = Replace Array Subset(array=w1757, new element #1=w1756, index #1=11 ("인덱스"), new element #2=w1755) -> (w1753:string[])  [unwired: 1 in]
                n505 = Build Array (concatenate)(w1761, w1753) -> (w1762:string[][])
              }
            }
          }
          n506 = call-poly "Data Classification.vi"("인덱스"=2, "DATA 입력"=w1616, "검색 문자열"=w1629) -> ("DATA 출력"=w1627:string[][])  [unwired: 4 in, 4 out]
          n507 = for {
            tunnel: w1609 -> [w1732] mode=indexing
            tunnel: [w1728] -> w1644 mode=indexing
            n508 = Index Array(array=w1732) -> (element #1=w1731:string, element #2=w1730:string)  [unwired: 2 in]
            n509 = call "Unit Conversion.vi"("환산단위"="kPa abs.", "입력단위"=w1730, "입력값"=w1731) -> ("환산값 (DBL)"=w1728:dbl)  [unwired: 3 in, 5 out]
          }
          n510 = for {
            tunnel: w1627 -> [w1710] mode=indexing
            tunnel: [w1709] -> w1626 mode=indexing
            tunnel: w1625 -> [w1714]
            n511 = Index Array(array=w1710, index #1=13 ("인덱스"), index #2=16 ("인덱스")) -> (element #1=w1712:string, element #2=w1705:string)
            n512 = call "Unit Conversion.vi"("환산단위"=w1714, "입력단위"=w1705, "입력값"=w1712) -> ("환산단위"=w1706:string, "환산값 (string)"=w1707:string)  [unwired: 3 in, 4 out]
            n513 = Replace Array Subset(array=w1710, new element #1=w1707, index #1=11 ("인덱스"), new element #2=w1706) -> (w1709:string[])  [unwired: 1 in]
          }
          n514 = Absolute Value(x=w1644) -> (abs(x)=w1639:dbl[])
          n515 = Fract/Exp String To Number(string=w1652) -> (number=w1654:dbl[])  [unwired: 3 in, 1 out]
          n516 = Array Max & Min(array=w1639) -> (max value=w1640:dbl)  [unwired: 3 out]
          n517 = Absolute Value(x=w1654) -> (abs(x)=w1637:dbl[])
          n518 = In Range and Coerce(upper limit=1000.0 ("상위 리미트"), x=w1640, lower limit=w1641) -> (In Range?=w1642:bool)  [unwired: 1 out]
          n519 = Array Max & Min(array=w1637) -> (max value=w1646:dbl)  [unwired: 3 out]
          n520 = case shown="거짓" w1642 {
            tunnel: [w1721 "kPa abs."] -> w1638
            tunnel: w1641 -> [w1726 _]
            tunnel: w1640 -> [w1725 _]
            frame False {
              n521 = Less?(x=w1725, y=w1726) -> (x < y?=w1724:bool)
              n522 = Select(t="Pa abs.", s=w1724, f="MPa abs.") -> (s? t:f=w1721:string)
            }
            frame True {
            }
          }
          n523 = call-poly "Data Sorting.vi"("기준열"=u16 11, "Data in"=w1626) -> ("Data out"=w1621:string[][])  [unwired: 8 in, 1 out]
          n524 = call-poly "Data Sorting.vi"("기준열"=w1645, "Data in"=w1657) -> ("Data out"=w1649:string[][])  [unwired: 8 in, 1 out]
          n525 = To Long Integer(number=w1645) -> (32bit integer=w1656:i32)
          n526 = Index Array(array=w1649, index (col)=w1656) -> (element=w1655:string[])  [unwired: 1 in]
          n527 = call-poly "Data Classification.vi"("인덱스"=2, "DATA 입력"=w1616, "검색 문자열"="DC Power Supply") -> ("행크기"=w1614:i32)  [unwired: 4 in, 4 out]
          n528 = Fract/Exp String To Number(string=w1655) -> (number=w1650:dbl[])  [unwired: 3 in, 1 out]
          n529 = Less Or Equal To 0?(x=w1614) -> (x <= 0?=w1613:bool)
          n530 = for {
            tunnel: w1646 -> [w1735]
            tunnel: w1649 -> [w1734] mode=indexing
            tunnel: w1650 -> [w1736] mode=indexing
            tunnel: [w1734] -> w1651 if=w1733
            stop <- w1733 stop-if-true
            n531 = Less Or Equal?(x=w1735, y=w1736) -> (x <= y?=w1733:bool)
          }
          n532 = Select(t="error" ("검색 문자열"), s=w1613, f="ok") -> (s? t:f=w1610:string)
          n533 = call "Variables Data IO.vi"("Select"=Cmd_Var_Data_IO."Resolution", "error in"=w1635, "Func_ext"=w1636) -> ("error out"=w1648:errorcluster, "Data Out"=w1660:string[][], "Func_ext Out"=w1647:string)  [unwired: 6 in]
          n534 = call "Calcu_STD Pressure_PC.vi"("STD 단위"=w1638, "Resolution"=w1660, "Cal STD (+)"=w1651, "Condition"=w1609) -> ("Data Out"=w1619:string[][], "STD Data"=w1620:string[][], "배열"=w1618:dbl[])  [unwired: 5 in]
          n535 = for {
            tunnel: [w1665] -> w1624 mode=indexing
            tunnel: w1621 -> [w1664]
            tunnel: w1618 -> [w1663] mode=indexing
            tunnel: w1610 -> [w1662]
            n536 = for {
              tunnel: [w1697] -> w1665
              tunnel: w1664 -> [w1695] mode=indexing
              tunnel: w1663 -> [w1678]
              tunnel: w1662 -> [w1666]
              stop <- w1703 stop-if-true
              n537 = Index Array(array=w1695, index #1=11 ("비활성화된 인덱스 (열)"), index #2=1 ("인덱스"), index #3=13 ("인덱스"), index #4=15 ("인덱스"), index #8=19 ("인덱스"), index #9=21 ("인덱스"), index #10=12 ("인덱스"), index #11=24 ("인덱스")) -> (element #1=w1676:string, element #2=w1674:string, element #3=w1672:string, element #4=w1670:string, element #5=w1669:string, element #6=w1680:string, element #7=w1679:string, element #8=w1701:string, element #9=w1691:string, element #10=w1668:string, element #11=w1688:string, element #12=w1687:string, element #13=w1693:string, element #14=w1692:string)  [unwired: 6 in]
              n538 = Fract/Exp String To Number(string=w1676) -> (number=w1704:dbl)  [unwired: 3 in, 1 out]
              n539 = call "Unit Conversion.vi"("환산단위"=w1668, "입력단위"=w1669, "입력값"=w1672) -> ("환산값 (string)"=w1681:string)  [unwired: 3 in, 5 out]
              n540 = call "Unit Conversion.vi"("환산단위"=w1668, "입력단위"=w1669, "입력값"=w1670) -> ("환산값 (string)"=w1667:string)  [unwired: 3 in, 5 out]
              n541 = call "Unit Conversion.vi"("환산단위"=w1668, "입력단위"=w1679, "입력값"=w1680) -> ("환산단위"=w1683:string, "환산값 (string)"=w1682:string)  [unwired: 3 in, 4 out]
              n542 = call "Unit Conversion.vi"("환산단위"=w1668, "입력단위"=w1691, "입력값"=w1701) -> ("환산단위"=w1696:string, "환산값 (string)"=w1698:string)  [unwired: 3 in, 4 out]
              n543 = call "Unit Conversion.vi"("환산단위"="실수", "입력단위"=w1687, "입력값"=w1688) -> ("환산단위"=w1684:string, "환산값 (string)"=w1685:string)  [unwired: 3 in, 4 out]
              n544 = call "Unit Conversion.vi"("환산단위"=w1668, "입력단위"=w1692, "입력값"=w1693) -> ("환산단위"=w1689:string, "환산값 (string)"=w1690:string)  [unwired: 3 in, 4 out]
              n545 = Less?(x=w1678, y=w1704) -> (x < y?=w1703:bool)
              n546 = Build Array(w1674, w1681, w1667, w1682, w1683, w1698, w1696, w1685, w1684, w1690, w1689, w1666) -> (w1697:string[])
            }
          }
          n547 = call "Variables Data IO.vi"("Select"=Cmd_Var_Data_IO."STD4", "error in"=w1648, "Data In"=w1624, "Func_ext"=w1647) -> ("error out"=w1623:errorcluster)  [unwired: 5 in, 2 out]
        }
        frame "20413-0" {
          w1772 = 11 ("인덱스")
          w1779 = 1.0 ("하위 리미트")
          w1783 = u16 11 ("기준열")
          w1792 = 0 ("인덱스 (행)")
          n548 = Index Array(array=w1769, index (col) #1=w1792, index (row) #2=w1792, index (col) #2=1 ("비활성화된 인덱스 (열)")) -> (element #1=w1791:string[], element #2=w1794:string)  [unwired: 1 in]
          n549 = for {
            tunnel: w1768 -> [w1817] mode=indexing
            tunnel: w1794 -> [w1814]
            shift-right: [w1819] -> w1787
            shift-left: string[][] [] -> [w1820]
            n550 = Index Array(array=w1817, index #1=13 ("인덱스"), index #2=16 ("인덱스"), index #3=2 ("인덱스")) -> (element #1=w1816:string, element #2=w1815:string, element #3=w1822:string)
            n551 = Equal?(x=w1822, y="Pressure Calibrator(-)") -> (x = y?=w1818:bool)
            n552 = case shown="참" w1818 {
              tunnel: w1817 -> [_ w1832]
              tunnel: [w1826 w1827] -> w1819
              tunnel: w1820 -> [w1826 w1836]
              tunnel: w1816 -> [_ w1835]
              tunnel: w1815 -> [_ w1834]
              tunnel: w1814 -> [_ w1833]
              frame False {
              }
              frame True {
                n553 = call "Unit Conversion.vi"("환산단위"=w1833, "입력단위"=w1834, "입력값"=w1835) -> ("환산단위"=w1830:string, "환산값 (string)"=w1831:string)  [unwired: 3 in, 4 out]
                n554 = Replace Array Subset(array=w1832, new element #1=w1831, index #1=11 ("인덱스"), new element #2=w1830) -> (w1828:string[])  [unwired: 1 in]
                n555 = Build Array (concatenate)(w1836, w1828) -> (w1827:string[][])
              }
            }
          }
          n556 = call "Variables Data IO.vi"("Select"=Cmd_Var_Data_IO."Resolution", "error in"=w1766, "Func_ext"=w1767) -> ("error out"=w1765:errorcluster, "Data Out"=w1796:string[][])  [unwired: 6 in, 1 out]
          n557 = for {
            tunnel: w1769 -> [w1809] mode=indexing
            tunnel: [w1805] -> w1782 mode=indexing
            n558 = Index Array(array=w1809) -> (element #1=w1808:string, element #2=w1807:string)  [unwired: 2 in]
            n559 = call "Unit Conversion.vi"("환산단위"="kPa", "입력단위"=w1807, "입력값"=w1808) -> ("환산값 (DBL)"=w1805:dbl)  [unwired: 3 in, 5 out]
          }
          n560 = Absolute Value(x=w1782) -> (abs(x)=w1777:dbl[])
          n561 = Array Max & Min(array=w1777) -> (max value=w1778:dbl)  [unwired: 3 out]
          n562 = Fract/Exp String To Number(string=w1791) -> (number=w1793:dbl[])  [unwired: 3 in, 1 out]
          n563 = In Range and Coerce(upper limit=1000.0 ("상위 리미트"), x=w1778, lower limit=w1779) -> (In Range?=w1780:bool)  [unwired: 1 out]
          n564 = Array Max & Min(array=w1793) -> (min value=w1784:dbl)  [unwired: 3 out]
          n565 = case shown="거짓" w1780 {
            tunnel: [w1798 "kPa"] -> w1776
            tunnel: w1779 -> [w1803 _]
            tunnel: w1778 -> [w1802 _]
            frame False {
              n566 = Less?(x=w1802, y=w1803) -> (x < y?=w1801:bool)
              n567 = Select(t="Pa", s=w1801, f="MPa") -> (s? t:f=w1798:string)
            }
            frame True {
            }
          }
          n568 = call-poly "Data Sorting.vi"("기준열"=w1783, "Data in"=w1787) -> ("Data out"=w1785:string[][])  [unwired: 8 in, 1 out]
          n569 = To Long Integer(number=w1783) -> (32bit integer=w1788:i32)
          n570 = Index Array(array=w1785, index (col)=w1788) -> (element=w1789:string[])  [unwired: 1 in]
          n571 = Fract/Exp String To Number(string=w1789) -> (number=w1786:dbl[])  [unwired: 3 in, 1 out]
          n572 = for {
            tunnel: w1784 -> [w1812]
            tunnel: w1785 -> [w1811] mode=indexing
            tunnel: w1786 -> [w1813] mode=indexing
            tunnel: [w1811] -> w1770 if=w1810
            stop <- w1810 stop-if-true
            n573 = Greater Or Equal?(x=w1812, y=w1813) -> (x >= y?=w1810:bool)
          }
          n574 = Index Array(array=w1770, index=w1772) -> (element=w1775:string)
          n575 = Search and Replace String(input string=w1775, search string="-" ("검색 문자열")) -> (result string=w1771:string)  [unwired: 6 in, 3 out]
          n576 = Replace Array Subset(array=w1770, new element=w1771, index=w1772) -> (w1773:string[])
          n577 = call "Calcu_STD Pressure_PC.vi"("STD 단위"=w1776, "Cal STD (-)"=w1770, "Resolution"=w1796, "Cal STD (+)"=w1773, "Condition"=w1769) -> ("Data Out"=w1764:string[][], "STD Data"=w1763:string[][])  [unwired: 4 in, 1 out]
        }
        frame "20414-0" {
          w1849 = 11 ("인덱스")
          w1856 = 1.0 ("하위 리미트")
          w1860 = u16 11 ("기준열")
          w1868 = 0 ("인덱스 (행)")
          n578 = Index Array(array=w1838) -> (element=w1837:string[])  [unwired: 2 in]
          n579 = Index Array(array=w1846, index (col) #1=w1868, index (row) #2=w1868, index (col) #2=1 ("비활성화된 인덱스 (열)")) -> (element #1=w1867:string[], element #2=w1870:string)  [unwired: 1 in]
          n580 = for {
            tunnel: w1845 -> [w1893] mode=indexing
            tunnel: w1870 -> [w1890]
            shift-right: [w1895] -> w1863
            shift-left: string[][] [] -> [w1896]
            n581 = Index Array(array=w1893, index #1=13 ("인덱스"), index #2=16 ("인덱스"), index #3=2 ("인덱스")) -> (element #1=w1892:string, element #2=w1891:string, element #3=w1898:string)
            n582 = Equal?(x=w1898, y="Pressure Calibrator(+)") -> (x = y?=w1894:bool)
            n583 = case shown="참" w1894 {
              tunnel: w1893 -> [_ w1908]
              tunnel: [w1902 w1903] -> w1895
              tunnel: w1896 -> [w1902 w1912]
              tunnel: w1892 -> [_ w1911]
              tunnel: w1891 -> [_ w1910]
              tunnel: w1890 -> [_ w1909]
              frame False {
              }
              frame True {
                n584 = call "Unit Conversion.vi"("환산단위"=w1909, "입력단위"=w1910, "입력값"=w1911) -> ("환산단위"=w1906:string, "환산값 (string)"=w1907:string)  [unwired: 3 in, 4 out]
                n585 = Replace Array Subset(array=w1908, new element #1=w1907, index #1=11 ("인덱스"), new element #2=w1906) -> (w1904:string[])  [unwired: 1 in]
                n586 = Build Array (concatenate)(w1912, w1904) -> (w1903:string[][])
              }
            }
          }
          n587 = call "Variables Data IO.vi"("Select"=Cmd_Var_Data_IO."Resolution", "error in"=w1843, "Func_ext"=w1844) -> ("error out"=w1842:errorcluster, "Data Out"=w1872:string[][])  [unwired: 6 in, 1 out]
          n588 = for {
            tunnel: w1846 -> [w1885] mode=indexing
            tunnel: [w1881] -> w1859 mode=indexing
            n589 = Index Array(array=w1885) -> (element #1=w1884:string, element #2=w1883:string)  [unwired: 2 in]
            n590 = call "Unit Conversion.vi"("환산단위"="kPa", "입력단위"=w1883, "입력값"=w1884) -> ("환산값 (DBL)"=w1881:dbl)  [unwired: 3 in, 5 out]
          }
          n591 = Absolute Value(x=w1859) -> (abs(x)=w1854:dbl[])
          n592 = Array Max & Min(array=w1854) -> (max value=w1855:dbl)  [unwired: 3 out]
          n593 = Fract/Exp String To Number(string=w1867) -> (number=w1869:dbl[])  [unwired: 3 in, 1 out]
          n594 = In Range and Coerce(upper limit=1000.0 ("상위 리미트"), x=w1855, lower limit=w1856) -> (In Range?=w1857:bool)  [unwired: 1 out]
          n595 = Array Max & Min(array=w1869) -> (max value=w1839:dbl)  [unwired: 3 out]
          n596 = case shown="거짓" w1857 {
            tunnel: [w1874 "kPa"] -> w1853
            tunnel: w1856 -> [w1879 _]
            tunnel: w1855 -> [w1878 _]
            frame False {
              n597 = Less?(x=w1878, y=w1879) -> (x < y?=w1877:bool)
              n598 = Select(t="Pa", s=w1877, f="MPa") -> (s? t:f=w1874:string)
            }
            frame True {
            }
          }
          n599 = call-poly "Data Sorting.vi"("기준열"=w1860, "Data in"=w1863) -> ("Data out"=w1861:string[][])  [unwired: 8 in, 1 out]
          n600 = To Long Integer(number=w1860) -> (32bit integer=w1864:i32)
          n601 = Index Array(array=w1861, index (col)=w1864) -> (element=w1865:string[])  [unwired: 1 in]
          n602 = Fract/Exp String To Number(string=w1865) -> (number=w1862:dbl[])  [unwired: 3 in, 1 out]
          n603 = for {
            tunnel: w1839 -> [w1888]
            tunnel: w1861 -> [w1887] mode=indexing
            tunnel: w1862 -> [w1889] mode=indexing
            tunnel: [w1887] -> w1847 if=w1886
            stop <- w1886 stop-if-true
            n604 = Less Or Equal?(x=w1888, y=w1889) -> (x <= y?=w1886:bool)
          }
          n605 = Index Array(array=w1847, index=w1849) -> (element=w1852:string)
          n606 = Search and Replace String(input string=w1852, search string="-" ("검색 문자열")) -> (result string=w1848:string)  [unwired: 6 in, 3 out]
          n607 = Replace Array Subset(array=w1847, new element=w1848, index=w1849) -> (w1850:string[])
          n608 = call "Calcu_STD Pressure_PC.vi"("STD 단위"=w1853, "Cal STD (-)"=w1837, "Resolution"=w1872, "Cal STD (+)"=w1850, "Condition"=w1846) -> ("Data Out"=w1841:string[][], "STD Data"=w1840:string[][])  [unwired: 4 in, 1 out]
        }
      }
      n609 = case shown="\"Pressure_2\"" w978 {
        tunnel: w980 -> [w989 w998]
        tunnel: [w988 w997] -> w979
        frame Default {
          n610 = for {
            tunnel: w989 -> [w996] mode=indexing
            tunnel: [w992] -> w988 mode=indexing
            n611 = Index Array(array=w996, index #1=1 ("인덱스"), index #2=3 ("인덱스")) -> (element #1=w994:string, element #2=w993:string)
            n612 = Format Into String(format string="%s %s" ("포맷 문자열"), w994, w993) -> (resulting string=w992:string)  [unwired: 2 in, 1 out]
          }
        }
        frame "Pressure_2" {
          n613 = for {
            tunnel: w998 -> [w1004] mode=indexing
            tunnel: [w1000] -> w997 mode=indexing
            n614 = Index Array(array=w1004, index #1=4 ("인덱스")) -> (element #1=w1002:string, element #2=w1001:string)  [unwired: 1 in]
            n615 = Format Into String(format string="%s %s" ("포맷 문자열"), w1002, w1001) -> (resulting string=w1000:string)  [unwired: 2 in, 1 out]
          }
        }
      }
    }
    frame "Resistance Meter" {
      n616 = case shown="\"Resistance Meter\", 기본" w1913 {
        tunnel: ["Resistance Source"] -> w1917
        tunnel: ["kΩ" ("환산단위")] -> w1916
        frame "Resistance Meter", Default {
        }
      }
      n617 = call-poly "Data Classification.vi"("인덱스"=2, "DATA 입력"=w1924, "검색 문자열"=w1917) -> ("DATA 출력"=w1919:string[][])  [unwired: 4 in, 4 out]
      n618 = for {
        tunnel: w1919 -> [w2005] mode=indexing
        tunnel: [w2000] -> w1918 mode=indexing
        tunnel: w1916 -> [w1995]
        n619 = Index Array(array=w2005, index #1=13 ("인덱스")) -> (element #1=w2006:string, element #2=w2004:string, element #3=w2002:string, element #4=w2003:string)  [unwired: 3 in]
        n620 = call "Unit Conversion.vi"("환산단위"=w1995, "입력단위"=w2003, "입력값"=w2006) -> ("환산값 (string)"=w1999:string)  [unwired: 3 in, 5 out]
        n621 = call "Unit Conversion.vi"("환산단위"=w1995, "입력단위"=w2003, "입력값"=w2004) -> ("환산값 (string)"=w1998:string)  [unwired: 3 in, 5 out]
        n622 = call "Unit Conversion.vi"("환산단위"=w1995, "입력단위"=w2003, "입력값"=w2002) -> ("환산단위"=w1996:string, "환산값 (string)"=w1997:string)  [unwired: 3 in, 4 out]
        n623 = Replace Array Subset(array=w2005, new element #1=w1999, index #1=13 ("인덱스"), new element #2=w1998, new element #3=w1997, new element #4=w1996) -> (w2000:string[])  [unwired: 3 in]
      }
      n624 = call-poly "Data Sorting.vi"("기준열"=u16 13, "error in (no error)"=w1923, "Data in"=w1918) -> ("error out"=w1921:errorcluster, "Data out"=w1915:string[][])  [unwired: 7 in]
      n625 = for {
        tunnel: w1915 -> [w1948]
        tunnel: w1922 -> [w1947] mode=indexing
        tunnel: [w1941] -> w1914 mode=indexing
        w1938 = 24 ("인덱스")
        w1939 = 21 ("인덱스")
        w1940 = 13 ("인덱스")
        n626 = Index Array(array=w1947) -> (element #3=w1944:string, element #4=w1946:string)  [unwired: 4 in, 2 out]
        n627 = Fract/Exp String To Number(string=w1944) -> (number=w1945:dbl)  [unwired: 3 in, 1 out]
        n628 = for {
          tunnel: w1948 -> [w1961] mode=indexing
          tunnel: w1946 -> [w1949]
          tunnel: [w1961] -> w1942
          tunnel: w1945 -> [w1977]
          tunnel: w1940 -> [w1960]
          tunnel: w1939 -> [w1964]
          tunnel: w1938 -> [w1963]
          tunnel: [w1962] -> w1943
          tunnel: [w1959] -> w1937
          tunnel: [w1958] -> w1936
          tunnel: [w1957] -> w1935
          tunnel: [w1956] -> w1934
          tunnel: [w1955] -> w1933
          tunnel: [w1954] -> w1932
          tunnel: [w1953] -> w1931
          tunnel: [w1952] -> w1930
          tunnel: [w1951] -> w1929
          tunnel: [w1950] -> w1928
          stop <- w1962 stop-if-true
          n629 = Index Array(array=w1961, index #1=w1960, index #8=w1964, index #9=w1963) -> (element #1=w1979:string, element #2=w1976:string, element #3=w1975:string, element #4=w1974:string, element #5=w1973:string, element #6=w1972:string, element #7=w1971:string, element #8=w1970:string, element #9=w1969:string, element #10=w1968:string, element #11=w1966:string, element #12=w1965:string)  [unwired: 9 in]
          n630 = call "Unit Conversion.vi"("환산단위"=w1949, "입력단위"=w1974, "입력값"=w1979) -> ("환산단위"=w1956:string, "환산값 (DBL)"=w1978:dbl, "환산값 (string)"=w1959:string)  [unwired: 3 in, 3 out]
          n631 = call "Unit Conversion.vi"("환산단위"=w1949, "입력단위"=w1974, "입력값"=w1976) -> ("환산값 (string)"=w1958:string)  [unwired: 3 in, 5 out]
          n632 = call "Unit Conversion.vi"("환산단위"=w1949, "입력단위"=w1974, "입력값"=w1975) -> ("환산값 (string)"=w1957:string)  [unwired: 3 in, 5 out]
          n633 = call "Unit Conversion.vi"("환산단위"=w1949, "입력단위"=w1972, "입력값"=w1973) -> ("환산값 (string)"=w1955:string)  [unwired: 3 in, 5 out]
          n634 = call "Unit Conversion.vi"("환산단위"=w1949, "입력단위"=w1970, "입력값"=w1971) -> ("환산값 (string)"=w1954:string)  [unwired: 3 in, 5 out]
          n635 = call "Unit Conversion.vi"("환산단위"="실수", "입력단위"=w1968, "입력값"=w1969) -> ("환산단위"=w1952:string, "환산값 (string)"=w1953:string)  [unwired: 3 in, 4 out]
          n636 = call "Unit Conversion.vi"("환산단위"=w1949, "입력단위"=w1965, "입력값"=w1966) -> ("환산단위"=w1950:string, "환산값 (string)"=w1951:string)  [unwired: 3 in, 4 out]
          n637 = Greater Or Equal?(x=w1978, y=w1977) -> (x >= y?=w1962:bool)
        }
        n638 = case shown="참" w1943 {
          tunnel: w1942 -> [_ w1994]
          tunnel: [_ w1993] -> w1941
          tunnel: w1940 -> [_ w1992]
          tunnel: w1937 -> [_ w1991]
          tunnel: w1936 -> [_ w1990]
          tunnel: w1935 -> [_ w1989]
          tunnel: w1934 -> [_ w1986]
          tunnel: w1933 -> [_ w1988]
          tunnel: w1932 -> [_ w1987]
          tunnel: w1931 -> [_ w1983]
          tunnel: w1939 -> [_ w1985]
          tunnel: w1930 -> [_ w1982]
          tunnel: w1938 -> [_ w1984]
          tunnel: w1929 -> [_ w1981]
          tunnel: w1928 -> [_ w1980]
          frame False {
          }
          frame True {
            n639 = Replace Array Subset(array=w1994, new element #1=w1991, index #1=w1992, new element #2=w1990, new element #3=w1989, new element #4=w1986, new element #5=w1988, new element #6=w1986, new element #7=w1987, new element #8=w1986, index #8=w1985, new element #9=w1983, index #9=w1984, new element #10=w1982, new element #11=w1981, new element #12=w1980) -> (w1993:string[])  [unwired: 9 in]
          }
        }
      }
    }
    frame "Torque_1" {
      w2037 = TRUE ("Write blank data ?(T)")
      w2042 = 0 ("비활성화된 인덱스 (열)")
      w2050 = 2 ("인덱스")
      n640 = call-poly "Data Classification.vi"("인덱스"=w2050, "DATA 입력"=w2052, "검색 문자열"="Torque Arm") -> ("DATA 출력"=w2035:string[][])  [unwired: 4 in, 4 out]
      n641 = call-poly "Data Classification.vi"("인덱스"=w2050, "DATA 입력"=w2052, "검색 문자열"="Dead Weight (Force)") -> ("DATA 출력"=w2048:string[][])  [unwired: 4 in, 4 out]
      n642 = for {
        tunnel: w2035 -> [w2075] mode=indexing
        tunnel: [w2072] -> w2034
        tunnel: [w2074] -> w2023 mode=indexing
        tunnel: [w2057] -> w2016
        tunnel: [w2056] -> w2019
        w2061 = "m" ("환산단위")
        n643 = Index Array(array=w2075, index #1=13 ("비활성화된 인덱스 (열)"), index #8=21 ("인덱스"), index #9=24 ("인덱스")) -> (element #1=w2083:string, element #2=w2081:string, element #3=w2080:string, element #4=w2079:string, element #5=w2078:string, element #6=w2077:string, element #7=w2076:string, element #8=w2066:string, element #9=w2063:string, element #10=w2062:string)  [unwired: 7 in]
        n644 = call "Unit Conversion.vi"("환산단위"=w2061, "입력단위"=w2079, "입력값"=w2083) -> ("환산값 (string)"=w2072:string)  [unwired: 3 in, 5 out]
        n645 = call "Unit Conversion.vi"("환산단위"=w2061, "입력단위"=w2079, "입력값"=w2081) -> ("환산값 (string)"=w2071:string)  [unwired: 3 in, 5 out]
        n646 = call "Unit Conversion.vi"("환산단위"=w2061, "입력단위"=w2079, "입력값"=w2080) -> ("환산단위"=w2058:string, "환산값 (DBL)"=w2057:dbl, "환산값 (string)"=w2070:string)  [unwired: 3 in, 3 out]
        n647 = call "Unit Conversion.vi"("환산단위"=w2061, "입력단위"=w2077, "입력값"=w2078) -> ("환산값 (string)"=w2069:string)  [unwired: 3 in, 5 out]
        n648 = call "Unit Conversion.vi"("환산단위"=w2061, "입력단위"=w2066, "입력값"=w2076) -> ("환산값 (string)"=w2068:string)  [unwired: 3 in, 5 out]
        n649 = call "Unit Conversion.vi"("환산단위"=w2061, "입력단위"=w2062, "입력값"=w2063) -> ("환산값 (DBL)"=w2056:dbl, "환산값 (string)"=w2059:string)  [unwired: 3 in, 4 out]
        n650 = Replace Array Subset(array=w2075, new element #1=w2072, index #1=13 ("인덱스"), new element #2=w2071, new element #3=w2070, new element #4=w2058, new element #5=w2069, new element #6=w2058, new element #7=w2068, new element #8=w2058, index #8=21 ("인덱스"), new element #9=w2059, index #9=24 ("인덱스"), new element #10=w2058) -> (w2074:string[])  [unwired: 7 in]
      }
      n651 = for {
        shift-right: [w2091] -> w2041
        shift-left: w2048 -> [w2092]
        tunnel: string[] ["Tare", "Tare_Push", "Tare_Pull"] -> [w2089] mode=indexing
        n652 = call-poly "Data Classification.vi"("삭제?(F)"=TRUE, "인덱스"=5, "DATA 입력"=w2092, "검색 문자열"=w2089) -> ("DATA 출력"=w2091:string[][])  [unwired: 3 in, 4 out]
      }
      n653 = Divide(x=w2019, y=2.0) -> (x/y=w2017:dbl)
      n654 = Add(x=w2016, y=w2017) -> (x+y=w2015:dbl)
      n655 = call "Create File Path.vi"("파일타입"=Cmd_File_Type."CSV", "항목"=Cmd_File_path."데이터파일경로", "에러 입력"=w2014, "문자열 in"="Torque Weight Set" ("delimiter (\\t)")) -> ("error out"=w2009:errorcluster, "파일경로"=w2010:path)  [unwired: 4 in, 2 out]
      n656 = call-poly <vilib>:"Read Delimited Spreadsheet.vi"("file path (dialog if empty)"=w2010, "delimiter (\\t)"="," ("delimiter (\\t)")) -> ("all rows"=w2008:string[][])  [unwired: 8 in, 5 out]
      n657 = Index Array(array=w2008, index (col)=w2042) -> (element=w2047:string[])  [unwired: 1 in]
      n658 = call-poly "Data Classification.vi"("인덱스"=2, "DATA 입력"=w2008, "검색 문자열"=w2034) -> ("DATA 출력"=w2044:string[][])  [unwired: 4 in, 4 out]
      n659 = call-poly "Array Deduplication.vi"("배열 in"=w2047) -> ("배열 out"=w2046:string[])  [unwired: 9 in, 1 out]
      n660 = for {
        tunnel: w2046 -> [w2086] mode=indexing
        tunnel: [w2087] -> w2043 mode=indexing
        tunnel: w2044 -> [w2085]
        tunnel: w2042 -> [w2084]
        n661 = call-poly "Data Classification.vi"("인덱스"=w2084, "DATA 입력"=w2085, "검색 문자열"=w2086) -> ("DATA 출력"=w2087:string[][])  [unwired: 4 in, 4 out]
      }
      n662 = call-poly "Data Sorting.vi"("기준열"=u16 3, "Data in"=w2023) -> ("Data out"=w2022:string[][])  [unwired: 8 in, 1 out]
      n663 = call "Variables Data IO.vi"("Select"=Cmd_Var_Data_IO."Resolution", "error in"=w2009, "Func_ext"=w2028) -> ("error out"=w2020:errorcluster, "Data Out"=w2030:string[][], "Func_ext Out"=w2027:string)  [unwired: 6 in]
      n664 = call "Calcu_Torque Weight.vi"("Resolution"=w2030, "Weight Set"=w2043, "torque arm"=w2015, "STD Data"=w2041, "Condition"=w2055) -> ("기타정보"=w2024:string[][], "Condition Out"=w2029:string[][], "분동조합"=w2032:string[][], "분동질량(kg)"=w2033:string[][])  [unwired: 3 in]
      n665 = Insert Into Array(array=w2022, new element=w2024) -> (w2021:string[][])  [unwired: 2 in]
      n666 = call "Variables Data IO.vi"("Write blank data ?(F)"=w2037, "Select"=Cmd_Var_Data_IO."STD3", "error in"=w2020, "Data In"=w2021, "Func_ext"=w2027) -> ("error out"=w2025:errorcluster, "Func_ext Out"=w2026:string)  [unwired: 4 in, 1 out]
      n667 = call "Variables Data IO.vi"("Write blank data ?(F)"=w2037, "Select"=Cmd_Var_Data_IO."STD2", "error in"=w2025, "Data In"=w2032, "Func_ext"=w2026) -> ("error out"=w2039:errorcluster)  [unwired: 4 in, 2 out]
    }
    frame "Torque_2" {
      w2095 = 3 ("인덱스")
      n668 = Index Array(array=w2125, index (col)=2 ("비활성화된 인덱스 (열)")) -> (element=w2122:string[])  [unwired: 1 in]
      n669 = call-poly "Data Classification.vi"("인덱스"=w2095, "DATA 입력"=w2128, "검색 문자열"="반시계방향") -> ("DATA 출력"=w2094:string[][])  [unwired: 4 in, 4 out]
      n670 = call-poly "Data Classification.vi"("인덱스"=w2095, "DATA 입력"=w2128, "검색 문자열"="시계방향") -> ("DATA 출력"=w2097:string[][])  [unwired: 4 in, 4 out]
      n671 = Fract/Exp String To Number(string=w2122) -> (number=w2121:dbl[])  [unwired: 3 in, 1 out]
      n672 = for {
        tunnel: w2121 -> [w2134] mode=indexing
        tunnel: w2097 -> [w2136]
        tunnel: [w2135] -> w2129 mode=indexing
        tunnel: w2094 -> [w2133]
        tunnel: [w2132] -> w2093 mode=indexing
        n673 = for {
          tunnel: w2136 -> [w2145] mode=indexing
          tunnel: [w2140] -> w2135
          tunnel: w2134 -> [w2148]
          tunnel: [w2138] -> w2132
          tunnel: w2133 -> [w2137] mode=indexing
          stop <- w2139 continue-if-true
          n674 = Index Array(array=w2145, index=13 ("인덱스")) -> (element=w2143:string)
          n675 = Fract/Exp String To Number(string=w2143) -> (number=w2142:dbl)  [unwired: 3 in, 1 out]
          n676 = Multiply(x=w2142, y=0.1) -> (x*y=w2141:dbl)
          n677 = Equal To 0?(x=w2148) -> (x = 0?=w2147:bool)
          n678 = In Range and Coerce(upper limit=w2142, x=w2148, lower limit=w2141) -> (In Range?=w2150:bool)  [unwired: 1 out]
          n679 = Or(x=w2147, y=w2150) -> (x .or. y?=w2149:bool)
          n680 = case shown="참" w2149 {
            tunnel: w2145 -> [_ w2152]
            tunnel: [_ w2152] -> w2140
            tunnel: [_ w2151] -> w2138
            tunnel: w2137 -> [_ w2151]
            frame False {
            }
            frame True {
            }
          }
          n681 = Empty Array?(array=w2140) -> (empty?=w2139:bool)
        }
      }
      n682 = call "Variables Data IO.vi"("Write blank data ?(F)"=TRUE ("Write blank data ?(T)"), "Select"=Cmd_Var_Data_IO."STD2", "error in"=w2127, "Data In"=w2093, "Func_ext"=w2124) -> ("error out"=w2100:errorcluster, "Func_ext Out"=w2099:string)  [unwired: 4 in, 1 out]
      n683 = global read "Global_Cal Info.vi" "Func List"() -> (w2107:string[][])
      n684 = global read "Global_Cal Info.vi" "Spec변경?"() -> (w2111:bool[])
      n685 = Index Array(array=w2107, index (col)=2 ("비활성화된 인덱스 (열)")) -> (element=w2109:string[])  [unwired: 1 in]
      n686 = Index Array(array=w2129, index (col)=25 ("인덱스 (행)")) -> (element=w2117:string[])  [unwired: 1 in]
      n687 = Search 1D Array(1D array=w2109, element=w2099) -> (index of element=w2110:i32)  [unwired: 1 in]
      n688 = for {
        tunnel: [w2130] -> w2114 mode=indexing
        tunnel: w2117 -> [w2131] mode=indexing
        n689 = Build Array(w2131, w2131, w2131) -> (w2130:string[])
      }
      n690 = Index Array(array=w2111, index=w2110) -> (element=w2106:bool)
      n691 = Select(t=Cmd_Var_Data_IO."Spec Old" ("Select"), s=w2106, f=Cmd_Var_Data_IO."Spec Default" ("Select")) -> (s? t:f=w2103:T1)
      n692 = call "Variables Data IO.vi"("Select"=w2103, "error in"=w2100, "Func_ext"=w2099) -> ("error out"=w2120:errorcluster, "Data Out"=w2116:string[][], "Func_ext Out"=w2118:string)  [unwired: 6 in]
      n693 = call "Spec Calculation.vi"("기준값 열번호"=2 ("열번호(기준값)"), "Resolution"=w2114, "Condition in"=w2125, "Spec Default"=w2116) -> ("Spec out"=w2112:string[][])  [unwired: 6 in, 1 out]
      n694 = call "Variables Data IO.vi"("Select"=Cmd_Var_Data_IO."Spec", "error in"=w2120, "Data In"=w2112, "Func_ext"=w2118) -> ("error out"=w2126:errorcluster)  [unwired: 5 in, 2 out]
    }
    frame Default {
      w2154 = string[][] [] ("Data out")
    }
  }
  "Cal STD" <- w27
  "Data Out" <- w33
  "Data Out 2" <- w5
  n695 = for {
    tunnel: w26 -> [w2159] mode=indexing
    tunnel: [w2156] -> w17 mode=indexing
    n696 = Concatenate Strings(w2159) -> (w2158:string)
    n697 = call <vilib>:"Trim Whitespace.vi"("string"=w2158) -> ("trimmed string"=w2157:string)  [unwired: 1 in]
    n698 = Empty String/Path?(string/path=w2157) -> (empty?=w2156:bool)
  }
  n699 = Empty Array?(array=w27) -> (empty?=w28:bool)
  "생성오류?" <- w28
  n700 = call "Variables Data IO.vi"("Write blank data ?(F)"=TRUE ("Write blank data ?(T)"), "Select"=Cmd_Var_Data_IO."STD1", "error in"=w36, "Data In"=w27, "Func_ext"=w2) -> ("error out"=→"error out":errorcluster, "Func_ext Out"=→"Func_ext Out":string)  [unwired: 4 in, 1 out]
  n701 = Or Array Elements(Boolean array=w17) -> (logical OR=w16:bool)
  "데이터오류?" <- w16
  n702 = Build Array(w28, w16) -> (w11:bool[])
  n703 = global read "Global_Cal Info.vi" "Func List"() -> (w15:string[][])
  n704 = global read "Global_Cal Info.vi" "std error?"() -> (w12:bool[][])
  n705 = Index Array(array=w15, index (col)=2 ("비활성화된 인덱스 (열)")) -> (element=w14:string[])  [unwired: 1 in]
  n706 = Search 1D Array(1D array=w14, element=w2) -> (index of element=w1:i32)  [unwired: 1 in]
  n707 = Replace Array Subset(array=w12, new element=w11, index (row)=w1) -> (w10:bool[][])  [unwired: 1 in]
  n708 = global write "Global_Cal Info.vi" "std error?"(w10) -> ()
